vi "Meas Process Config Panel.vi"(8 "error in (no error)":errorcluster, 11 "session in":T4={"adc"={"niScope"={"channel cfg"=[], "sessions"=[], "multi cards"=FALSE, "channels"=0, "type"=enum."n/a", "memory [B/chn]"=0, "ext. clock [Hz]"=0.0, "samples count"=0, "use streaming"=FALSE, "proc setup"={"packet size [smpl]"=0, "current timeout [s]"=0.0, "blk2blk timeout [s]"=0.0, "event time"=timestamp(0 s since 1904-01-01), "temp sampl T [s]"=0.0, "data queue"=refnum, "stop notifier"=refnum, "proc ref"=refnum}, "sample width [B]"=0, "ranges [V]"=[], "trigger setup"={"coupling"=1, "level [V]"=0.0, "slope"=0, "mode"=enum."Immediate", "pre-trigger [%]"=0.0}, "fs [Hz]"=0.0, "bitres [bit]"=0, "clock source"=enum."VAL_NO_SOURCE"}, "3458A"={"channels"=[], "sync unit"={"VISA"="", "type"=enum."Picotest U6200A"}, "awg unit"={"type"=enum."Agilent 331xxA to 332xxA", "VISA"="", "enable 10MHz ref"=FALSE, "cmi ckd2"={"VISA"="", "clock source"=enum."Auto", "manual ref clk"=FALSE, "ref clock [Hz]"=0.0, "div mode"=enum."Set divisor directly"}, "cmi sync v3"={"VISA"="", "baud rate [bd/s]"=115200, "source"=enum."Auto", "hv range"=enum."1kV", "fsrc is fixed"=FALSE, "fsrc [Hz]"=10000000.0, "freq integ [s]"=1.0, "freq filter"=5, "trig level"=enum."TTL 5V", "chn1 mode"=enum."Source divider", "chn1 level"=enum."Positive 5V", "chn2 mode"=enum."Source divider", "chn2 level"=enum."Positive 5V", "chn2 div"=1, "chn3 mode"=enum."Chn 1 Active", "chn3 level"=enum."Positive 5V", "chn1 div entry"=enum."Calculate nearest divisor from measured fx", "chn1 dev limit [%]"=1.0, "chn1 check dev"=FALSE}, "trigger"={"source"=enum."Immediate", "slope"=enum."POS", "coupling"=enum."DC", "level [V]"=0.0, "hysteresis [V]"=0.0, "pre-trigger [%]"=0.0}, "HMF2500 cfg"={"Baud Rate"=9600, "Parity"=0, "Data Bits"=8, "Flow Control"=4}}, "sync mode"=enum."MASTER-SLAVE, MASTER clocked by TIMER", "streaming mode"=FALSE, "idn mode"=enum."Auto", "sampling mode"=enum."DCV", "sample memory [B]"=0, "proc setup"={"channel id"=0, "packet size [smpl]"=0, "current timeout [s]"=0.0, "blk2blk timeout [s]"=0.0, "event time"=timestamp(0 s since 1904-01-01), "stop notifier"=refnum, "data queues"=[], "proc refs"=[], "bus semaphore"=refnum}, "sample size [B]"=0, "sample count"=0, "aux data"={"channel id"=0, "valid?"=[], "gain [V]"=[], "timestamp [s]"=[], "Ts [s]"=0.0, "abs timestamp"=timestamp(0 s since 1904-01-01), "t [deg C]"=[], "multiplex timestamp [s]"=-1.0, "only multiplex?"=FALSE, "multiplex smpl offset"=0, "overflow?"=FALSE}, "ranges [V]"=[], "aperture [s]"=0.0, "LEVEL trigger"={"edge"=enum."POS", "level [V]"=0.0, "coupling"=enum."DC"}, "trigger mode"=enum."AUTO", "measure temp.?"=FALSE, "disp mesages"=[], "shared bus?"=FALSE, "disable display?"=FALSE, "aper mode"=enum."Manual", "aper rules"=[], "multiplex"={"cycles"=0, "delay [s]"=0.0, "enabled"=FALSE, "overhead [s]"=1.0, "tot smpls"=0, "sub-rec"=0, "overhead [%]"=0.0, "emulated"=FALSE}, "F8588 lpf"=enum."Off", "F8588 pll"=enum."Off", "F8588 couple"=enum."DC, auto", "fs"={"freq mode"=enum."fs or Ts", "fs [Hz]"=0.0, "fref [Hz]"=0.0, "mul"=0.0, "div"=0.0}, "fs mode"=enum."fs or Ts", "init timestamp"=timestamp(0 s since 1904-01-01), "last report timestamp"=timestamp(0 s since 1904-01-01)}, "dsdll"={"dsdll"={"dsdll path"=path "", "dsdll handle"=[], "output devices"=[], "capture devices"=[]}, "channels"=0, "device id"=0, "channel idns"=[], "proc setup"={"packet size [smpl]"=0, "current timeout [s]"=0.0, "blk2blk timeout [s]"=0.0, "event time"=timestamp(0 s since 1904-01-01), "data queue"=refnum, "stop notifier"=refnum, "proc ref"=refnum}, "samples count"=0, "fs [Hz]"=0.0}, "type"=enum."niScope", "channel idn str"=[], "aux instr idn str"=[], "modified?"=FALSE, "simadc"={"channels"=[], "range [V]"=0.0, "Ts step [s]"=0.0, "time [s]"=0.0, "fs [Hz]"=0.0, "count"=0, "smpl offset"=0, "set count"=0, "bit res"=0}, "force rst?"=FALSE, "exit mode"=enum."Immediate reset", "exit dly"=0.0, "exit tmr"=timestamp(0 s since 1904-01-01), "busy?"=FALSE, "accessed?"=FALSE, "multiplex"={"Type"=enum."Dummy", "gen com ssn"={"visa"="", "primary"=enum."None", "secondary"=enum."None", "channels"=[]}, "delay before [s]"=0.0, "delay post [s]"=0.0, "sequence"=[], "enabled"=FALSE, "ref timestamp [s]"=0.0, "idn string"="", "dev niScope"="", "niScope idx"=0, "QPMX ssn"={"visa"="", "switch mode"=enum."Switched by TWM", "sequence"=[], "timing delays"=[], "polarity"=enum."Positive", "ss delay (s)"=2.0, "internal timer (s)"=1.0, "Last loaded sequence file"=path "", "startup delay (s)"=2.0}, "VISA mux ssn"={"VISA"="", "paths"=[], "idn command"="", "serial cfg"={"Baud rate"=9600, "Data bits"=8, "Parity"=0, "Stop bits"=10, "Flow control"=0, "End Mode Read"=enum."None", "End Mode Write"=enum."None", "Term character"=0, "Term enable"=FALSE}}}, "keysight dso"={"VISA"="", "channels"=[], "bw limit [Hz]"=0.0, "resolution"=enum."Basic", "trig noise reject"=enum."Normal", "N"=0, "trigger config"={"trigger source"=enum."Immediate", "trigger slope"=enum."Negative", "level [V]"=0.0, "hysteresis [V]"=0.001, "pre-trig [%]"=50}, "fs [Hz]"=0.0, "timeout stop"=timestamp(0 s since 1904-01-01), "waiting for opc"=FALSE, "fetch offset [smpl]"=0, "abs timestamp"=timestamp(0 s since 1904-01-01), "ranges [V]"=[], "decimation"=1.0, "ext ref"=FALSE, "emulate aperture"=FALSE, "model"=enum."DSO91304"}, "cdaq"={"mclk [Hz]"=12800000.0, "ADC task"="", "mclk reference"="", "fs [Hz]"=50000.0, "queue adc cmd"=refnum, "queue adc data"=refnum, "adc proc ref"=refnum, "channels"=[], "last channels"=[], "timeout"=timestamp(0 s since 1904-01-01), "N"=1000, "mclk mode"=enum."Free running", "ext mclk source"=""}, "ignore overload"=FALSE, "ADS127L21"={"VISA"="", "chn list"=[], "record size"=0, "phys. channels"=0, "adc fifo size"=0, "channels"=[], "ext refclk?"=FALSE, "fs [Hz]"=0.0, "ext refclk [Hz]"=0.0, "meas refclk [Hz]"=0.0, "EXTOUT mode"=enum."ADCCLK", "EXTOUT polarity"=enum."NORM", "EXTOUT divisor"=0}}, "sequence"=[], "sequence setup"={"group setups"=[], "rec count"=0, "range mode"=enum."Keep defaults", "fs mode"=enum."Frequency", "rng even"=0.0, "rng odd"=0.0, "folder"=path "", "name base"="", "meas id"=0, "settle [s]"=0.0, "comment"="", "avg count"=0, "fs-abs-fr fr"=0.0, "fs-abs-fr fs"=0.0, "fs-div fr"=0.0, "fs-div div"=0.0, "fs-mn fr"=0.0, "fs-mn mul"=0.0, "fs-mn div"=0.0, "fs-rat fr"=0.0, "fs-rat rat"=0.0}, "golpi"=refnum, "processing setup"={"mode"=enum."Raw", "call after avgs?"=FALSE, "calculate?"=FALSE, "raw mode"={"command"="", "result mode"=enum."Display console output (only Octave)", "res variable"=""}, "QWTB"={"QWTB path"=path "", "alg filter path"="", "alg ids"=[], "alg parameters"=[], "parsed parameters"=[], "selected alg id"="", "selected unc mode"=enum."None", "qwtb mcc"=100, "qwtb timeout"=90, "qwtb covg"=95.0, "qwtb ofs"=0, "qwtb lim data"=0, "multicore"={"jobs folder"=path "", "cores"=0, "max jobs"=0, "mode"=enum."Singlecore"}, "unc once?"=FALSE, "qwtb tstemp"=enum."Enabled (default)", "octave reset"=FALSE, "exec mode"=enum."Single-core"}}, "corrections"={"transducers"={"channels"=[], "last path"=path "", "root path"=path ""}, "digitizer"={"last path"=path "", "channel paths"=[], "channel idns"=[], "correction name"="", "channel names"=[], "folders to copy"=[], "channel valid"=[], "correction path"=path "", "correction rel path"="", "rel folders to copy"=[], "root path"=path ""}}, "assist cfg"={"P"=0, "Q"=0, "rel shift"=0.0, "ref freq"=0.0, "min fs"=0.0, "max fs tol"=0.0, "min int"=0.0, "max int"=0.0, "max err"=0.0, "max timeout"=0.0}} {"corrections"."transducers"."channels"."Phase index" min=1 step=1; "adc"."ADS127L21"."channels"."Channel" min=1 max=8 step=1; "adc"."ADS127L21"."channels"."Range [Vpk]" items=["±1.65V", "±2V"]; "adc"."cdaq"."last channels"."Channel id" min=0 step=1; "adc"."cdaq"."channels"."Channel id" min=0 step=1; "adc"."keysight dso"."decimation" min=1.0; "adc"."keysight dso"."bw limit [Hz]" format="%#_6p"; "adc"."keysight dso"."channels"."Offset [V]" format="%#_6p"; "adc"."keysight dso"."channels"."Range [Vpk]" min=0.0 format="%#_6p"; "adc"."keysight dso"."channels"."Channel" min=1; "adc"."multiplex"."VISA mux ssn"."serial cfg"."Flow control" items=["None", "XON/XOFF", "CTS/RTS", "XON/XOFF + CTS/RTS", "DTR/DSR", "XON/XOFF + DTR/DSR"]; "adc"."multiplex"."VISA mux ssn"."serial cfg"."Stop bits" items=["1 bit"=10, "1.5 bits"=15, "2 bits"=20]; "adc"."multiplex"."VISA mux ssn"."serial cfg"."Parity" items=["None", "Odd", "Even", "Mark", "Space"]; "adc"."multiplex"."VISA mux ssn"."serial cfg"."Data bits" items=["5 bits"=5, "6 bits"=6, "7 bits"=7, "8 bits"=8]; "adc"."multiplex"."VISA mux ssn"."serial cfg"."Baud rate" items=["150 Bd"=150, "300 Bd"=300, "600 Bd"=600, "1200 Bd"=1200, "2400 Bd"=2400, "4800 Bd"=4800, "9600 Bd"=9600, "19.2 kBd"=19200, "38.4 kBd"=38400, "57.6 kBd"=57600, "115.2 kBd"=115200]; "adc"."multiplex"."QPMX ssn"."startup delay (s)" min=0.0 step=1.0; "adc"."multiplex"."QPMX ssn"."internal timer (s)" min=0.0 step=1.0; "adc"."multiplex"."QPMX ssn"."ss delay (s)" min=0.0 step=1.0; "adc"."multiplex"."QPMX ssn"."timing delays" min=1 max=255 step=1; "adc"."3458A"."awg unit"."HMF2500 cfg"."Flow Control" items=["None", "XON/XOFF", "RTS/CTS", "XON/XOFF & RTS/CTS", "DTR/DSR", "XON/XOFF & DTR/DSR"]; "adc"."3458A"."awg unit"."HMF2500 cfg"."Data Bits" items=["7"=7, "8"=8]; "adc"."3458A"."awg unit"."HMF2500 cfg"."Parity" items=["None", "Odd", "Even", "Mark", "Space"]; "adc"."3458A"."awg unit"."HMF2500 cfg"."Baud Rate" items=["300"=300, "600"=600, "1200"=1200, "2400"=2400, "4800"=4800, "9600"=9600, "19200"=19200]; "adc"."3458A"."awg unit"."cmi sync v3"."chn2 div" min=1 max=100000000 step=1; "adc"."3458A"."awg unit"."cmi sync v3"."fsrc [Hz]" format="%_8p"; "adc"."3458A"."channels"."Range [Vpk]" min=0.0; "adc"."niScope"."trigger setup"."pre-trigger [%]" format="%.2f"; "adc"."niScope"."trigger setup"."level [V]" format="%.2f"; "adc"."niScope"."trigger setup"."coupling" items=["AC"=0, "DC"=1, "HF Reject"=3, "LF Reject"=4, "AC Plus HF Reject"=1001]; "adc"."niScope"."channel cfg"."Range [Vpk]" min=0.0; "adc"."niScope"."channel cfg"."Channel" min=0}) -> (0 "error out":errorcluster, 3 "session out":T4={"adc"={"niScope"={"channel cfg"=[], "sessions"=[], "multi cards"=FALSE, "channels"=0, "type"=enum."n/a", "memory [B/chn]"=0, "ext. clock [Hz]"=0.0, "samples count"=0, "use streaming"=FALSE, "proc setup"={"packet size [smpl]"=0, "current timeout [s]"=0.0, "blk2blk timeout [s]"=0.0, "event time"=timestamp(0 s since 1904-01-01), "temp sampl T [s]"=0.0, "data queue"=refnum, "stop notifier"=refnum, "proc ref"=refnum}, "sample width [B]"=0, "ranges [V]"=[], "trigger setup"={"coupling"=1, "level [V]"=0.0, "slope"=0, "mode"=enum."Immediate", "pre-trigger [%]"=0.0}, "fs [Hz]"=0.0, "bitres [bit]"=0, "clock source"=enum."VAL_NO_SOURCE"}, "3458A"={"channels"=[], "sync unit"={"VISA"="", "type"=enum."Picotest U6200A"}, "awg unit"={"type"=enum."Agilent 331xxA to 332xxA", "VISA"="", "enable 10MHz ref"=FALSE, "cmi ckd2"={"VISA"="", "clock source"=enum."Auto", "manual ref clk"=FALSE, "ref clock [Hz]"=0.0, "div mode"=enum."Set divisor directly"}, "cmi sync v3"={"VISA"="", "baud rate [bd/s]"=115200, "source"=enum."Auto", "hv range"=enum."1kV", "fsrc is fixed"=FALSE, "fsrc [Hz]"=10000000.0, "freq integ [s]"=1.0, "freq filter"=5, "trig level"=enum."TTL 5V", "chn1 mode"=enum."Source divider", "chn1 level"=enum."Positive 5V", "chn2 mode"=enum."Source divider", "chn2 level"=enum."Positive 5V", "chn2 div"=1, "chn3 mode"=enum."Chn 1 Active", "chn3 level"=enum."Positive 5V", "chn1 div entry"=enum."Calculate nearest divisor from measured fx", "chn1 dev limit [%]"=1.0, "chn1 check dev"=FALSE}, "trigger"={"source"=enum."Immediate", "slope"=enum."POS", "coupling"=enum."DC", "level [V]"=0.0, "hysteresis [V]"=0.0, "pre-trigger [%]"=0.0}, "HMF2500 cfg"={"Baud Rate"=9600, "Parity"=0, "Data Bits"=8, "Flow Control"=4}}, "sync mode"=enum."MASTER-SLAVE, MASTER clocked by TIMER", "streaming mode"=FALSE, "idn mode"=enum."Auto", "sampling mode"=enum."DCV", "sample memory [B]"=0, "proc setup"={"channel id"=0, "packet size [smpl]"=0, "current timeout [s]"=0.0, "blk2blk timeout [s]"=0.0, "event time"=timestamp(0 s since 1904-01-01), "stop notifier"=refnum, "data queues"=[], "proc refs"=[], "bus semaphore"=refnum}, "sample size [B]"=0, "sample count"=0, "aux data"={"channel id"=0, "valid?"=[], "gain [V]"=[], "timestamp [s]"=[], "Ts [s]"=0.0, "abs timestamp"=timestamp(0 s since 1904-01-01), "t [deg C]"=[], "multiplex timestamp [s]"=-1.0, "only multiplex?"=FALSE, "multiplex smpl offset"=0, "overflow?"=FALSE}, "ranges [V]"=[], "aperture [s]"=0.0, "LEVEL trigger"={"edge"=enum."POS", "level [V]"=0.0, "coupling"=enum."DC"}, "trigger mode"=enum."AUTO", "measure temp.?"=FALSE, "disp mesages"=[], "shared bus?"=FALSE, "disable display?"=FALSE, "aper mode"=enum."Manual", "aper rules"=[], "multiplex"={"cycles"=0, "delay [s]"=0.0, "enabled"=FALSE, "overhead [s]"=1.0, "tot smpls"=0, "sub-rec"=0, "overhead [%]"=0.0, "emulated"=FALSE}, "F8588 lpf"=enum."Off", "F8588 pll"=enum."Off", "F8588 couple"=enum."DC, auto", "fs"={"freq mode"=enum."fs or Ts", "fs [Hz]"=0.0, "fref [Hz]"=0.0, "mul"=0.0, "div"=0.0}, "fs mode"=enum."fs or Ts", "init timestamp"=timestamp(0 s since 1904-01-01), "last report timestamp"=timestamp(0 s since 1904-01-01)}, "dsdll"={"dsdll"={"dsdll path"=path "", "dsdll handle"=[], "output devices"=[], "capture devices"=[]}, "channels"=0, "device id"=0, "channel idns"=[], "proc setup"={"packet size [smpl]"=0, "current timeout [s]"=0.0, "blk2blk timeout [s]"=0.0, "event time"=timestamp(0 s since 1904-01-01), "data queue"=refnum, "stop notifier"=refnum, "proc ref"=refnum}, "samples count"=0, "fs [Hz]"=0.0}, "type"=enum."niScope", "channel idn str"=[], "aux instr idn str"=[], "modified?"=FALSE, "simadc"={"channels"=[], "range [V]"=0.0, "Ts step [s]"=0.0, "time [s]"=0.0, "fs [Hz]"=0.0, "count"=0, "smpl offset"=0, "set count"=0, "bit res"=0}, "force rst?"=FALSE, "exit mode"=enum."Immediate reset", "exit dly"=0.0, "exit tmr"=timestamp(0 s since 1904-01-01), "busy?"=FALSE, "accessed?"=FALSE, "multiplex"={"Type"=enum."Dummy", "gen com ssn"={"visa"="", "primary"=enum."None", "secondary"=enum."None", "channels"=[]}, "delay before [s]"=0.0, "delay post [s]"=0.0, "sequence"=[], "enabled"=FALSE, "ref timestamp [s]"=0.0, "idn string"="", "dev niScope"="", "niScope idx"=0, "QPMX ssn"={"visa"="", "switch mode"=enum."Switched by TWM", "sequence"=[], "timing delays"=[], "polarity"=enum."Positive", "ss delay (s)"=2.0, "internal timer (s)"=1.0, "Last loaded sequence file"=path "", "startup delay (s)"=2.0}, "VISA mux ssn"={"VISA"="", "paths"=[], "idn command"="", "serial cfg"={"Baud rate"=9600, "Data bits"=8, "Parity"=0, "Stop bits"=10, "Flow control"=0, "End Mode Read"=enum."None", "End Mode Write"=enum."None", "Term character"=0, "Term enable"=FALSE}}}, "keysight dso"={"VISA"="", "channels"=[], "bw limit [Hz]"=0.0, "resolution"=enum."Basic", "trig noise reject"=enum."Normal", "N"=0, "trigger config"={"trigger source"=enum."Immediate", "trigger slope"=enum."Negative", "level [V]"=0.0, "hysteresis [V]"=0.001, "pre-trig [%]"=50}, "fs [Hz]"=0.0, "timeout stop"=timestamp(0 s since 1904-01-01), "waiting for opc"=FALSE, "fetch offset [smpl]"=0, "abs timestamp"=timestamp(0 s since 1904-01-01), "ranges [V]"=[], "decimation"=1.0, "ext ref"=FALSE, "emulate aperture"=FALSE, "model"=enum."DSO91304"}, "cdaq"={"mclk [Hz]"=12800000.0, "ADC task"="", "mclk reference"="", "fs [Hz]"=50000.0, "queue adc cmd"=refnum, "queue adc data"=refnum, "adc proc ref"=refnum, "channels"=[], "last channels"=[], "timeout"=timestamp(0 s since 1904-01-01), "N"=1000, "mclk mode"=enum."Free running", "ext mclk source"=""}, "ignore overload"=FALSE, "ADS127L21"={"VISA"="", "chn list"=[], "record size"=0, "phys. channels"=0, "adc fifo size"=0, "channels"=[], "ext refclk?"=FALSE, "fs [Hz]"=0.0, "ext refclk [Hz]"=0.0, "meas refclk [Hz]"=0.0, "EXTOUT mode"=enum."ADCCLK", "EXTOUT polarity"=enum."NORM", "EXTOUT divisor"=0}}, "sequence"=[], "sequence setup"={"group setups"=[], "rec count"=0, "range mode"=enum."Keep defaults", "fs mode"=enum."Frequency", "rng even"=0.0, "rng odd"=0.0, "folder"=path "", "name base"="", "meas id"=0, "settle [s]"=0.0, "comment"="", "avg count"=0, "fs-abs-fr fr"=0.0, "fs-abs-fr fs"=0.0, "fs-div fr"=0.0, "fs-div div"=0.0, "fs-mn fr"=0.0, "fs-mn mul"=0.0, "fs-mn div"=0.0, "fs-rat fr"=0.0, "fs-rat rat"=0.0}, "golpi"=refnum, "processing setup"={"mode"=enum."Raw", "call after avgs?"=FALSE, "calculate?"=FALSE, "raw mode"={"command"="", "result mode"=enum."Display console output (only Octave)", "res variable"=""}, "QWTB"={"QWTB path"=path "", "alg filter path"="", "alg ids"=[], "alg parameters"=[], "parsed parameters"=[], "selected alg id"="", "selected unc mode"=enum."None", "qwtb mcc"=100, "qwtb timeout"=90, "qwtb covg"=95.0, "qwtb ofs"=0, "qwtb lim data"=0, "multicore"={"jobs folder"=path "", "cores"=0, "max jobs"=0, "mode"=enum."Singlecore"}, "unc once?"=FALSE, "qwtb tstemp"=enum."Enabled (default)", "octave reset"=FALSE, "exec mode"=enum."Single-core"}}, "corrections"={"transducers"={"channels"=[], "last path"=path "", "root path"=path ""}, "digitizer"={"last path"=path "", "channel paths"=[], "channel idns"=[], "correction name"="", "channel names"=[], "folders to copy"=[], "channel valid"=[], "correction path"=path "", "correction rel path"="", "rel folders to copy"=[], "root path"=path ""}}, "assist cfg"={"P"=0, "Q"=0, "rel shift"=0.0, "ref freq"=0.0, "min fs"=0.0, "max fs tol"=0.0, "min int"=0.0, "max int"=0.0, "max err"=0.0, "max timeout"=0.0}} {"corrections"."transducers"."channels"."Phase index" min=1 step=1; "adc"."ADS127L21"."channels"."Channel" min=1 max=8 step=1; "adc"."ADS127L21"."channels"."Range [Vpk]" items=["±1.65V", "±2V"]; "adc"."cdaq"."last channels"."Channel id" min=0 step=1; "adc"."cdaq"."channels"."Channel id" min=0 step=1; "adc"."keysight dso"."decimation" min=1.0; "adc"."keysight dso"."bw limit [Hz]" format="%#_6p"; "adc"."keysight dso"."channels"."Offset [V]" format="%#_6p"; "adc"."keysight dso"."channels"."Range [Vpk]" min=0.0 format="%#_6p"; "adc"."keysight dso"."channels"."Channel" min=1; "adc"."multiplex"."VISA mux ssn"."serial cfg"."Flow control" items=["None", "XON/XOFF", "CTS/RTS", "XON/XOFF + CTS/RTS", "DTR/DSR", "XON/XOFF + DTR/DSR"]; "adc"."multiplex"."VISA mux ssn"."serial cfg"."Stop bits" items=["1 bit"=10, "1.5 bits"=15, "2 bits"=20]; "adc"."multiplex"."VISA mux ssn"."serial cfg"."Parity" items=["None", "Odd", "Even", "Mark", "Space"]; "adc"."multiplex"."VISA mux ssn"."serial cfg"."Data bits" items=["5 bits"=5, "6 bits"=6, "7 bits"=7, "8 bits"=8]; "adc"."multiplex"."VISA mux ssn"."serial cfg"."Baud rate" items=["150 Bd"=150, "300 Bd"=300, "600 Bd"=600, "1200 Bd"=1200, "2400 Bd"=2400, "4800 Bd"=4800, "9600 Bd"=9600, "19.2 kBd"=19200, "38.4 kBd"=38400, "57.6 kBd"=57600, "115.2 kBd"=115200]; "adc"."multiplex"."QPMX ssn"."startup delay (s)" min=0.0 step=1.0; "adc"."multiplex"."QPMX ssn"."internal timer (s)" min=0.0 step=1.0; "adc"."multiplex"."QPMX ssn"."ss delay (s)" min=0.0 step=1.0; "adc"."multiplex"."QPMX ssn"."timing delays" min=1 max=255 step=1; "adc"."3458A"."awg unit"."HMF2500 cfg"."Flow Control" items=["None", "XON/XOFF", "RTS/CTS", "XON/XOFF & RTS/CTS", "DTR/DSR", "XON/XOFF & DTR/DSR"]; "adc"."3458A"."awg unit"."HMF2500 cfg"."Data Bits" items=["7"=7, "8"=8]; "adc"."3458A"."awg unit"."HMF2500 cfg"."Parity" items=["None", "Odd", "Even", "Mark", "Space"]; "adc"."3458A"."awg unit"."HMF2500 cfg"."Baud Rate" items=["300"=300, "600"=600, "1200"=1200, "2400"=2400, "4800"=4800, "9600"=9600, "19200"=19200]; "adc"."3458A"."awg unit"."cmi sync v3"."chn2 div" min=1 max=100000000 step=1; "adc"."3458A"."awg unit"."cmi sync v3"."fsrc [Hz]" format="%_8p"; "adc"."3458A"."channels"."Range [Vpk]" min=0.0; "adc"."niScope"."trigger setup"."pre-trigger [%]" format="%.2f"; "adc"."niScope"."trigger setup"."level [V]" format="%.2f"; "adc"."niScope"."trigger setup"."coupling" items=["AC"=0, "DC"=1, "HF Reject"=3, "LF Reject"=4, "AC Plus HF Reject"=1001]; "adc"."niScope"."channel cfg"."Range [Vpk]" min=0.0; "adc"."niScope"."channel cfg"."Channel" min=0})   [LabVIEW 2020]
doc: "Configuration panel for result calculator. Select tab to select method of calculation."
uses:
  Meas Session.ctl
  adc/ADC Session.ctl
  drivers/niScope/niScope Session.ctl
  drivers/niScope/niScope Virtual Channel Config.ctl
  drivers/niScope/niScope Virtual Channel Mode.ctl
  drivers/niScope/niScope Virtual Channel Input Z.ctl
  drivers/niScope/niScope Virtual Channel Coupling.ctl
  drivers/niScope/niScope Type.ctl
  drivers/niScope/niScope Digitizing Process Options.ctl
  drivers/niScope/niScope Data Packet.ctl
  drivers/niScope/niScope Trigger Setup.ctl
  <instrlib>/niScope/Controls/niScope trigger coupling.ctl
  <instrlib>/niScope/Controls/niScope trigger slope.ctl
  drivers/niScope/niScope Reference Clock.ctl
  drivers/DMM/3458A Digitizer Session.ctl
  drivers/DMM/3458A Virtual Channel Config.ctl
  drivers/Counter/Counter Session.ctl
  drivers/Counter/Counter Type.ctl
  drivers/AWG/AWG Session.ctl
  drivers/AWG/AWG Type.ctl
  drivers/AWG/CMI Clock Divider v2/CMI ckd2 Session.ctl
  drivers/AWG/CMI Clock Divider v2/CMI ckd2 Source Mode.ctl
  drivers/AWG/CMI Clock Divider v2/CMI ckd2 Divisor Mode.ctl
  drivers/AWG/CMI Sync V3/CMI Sync V3 session.ctl
  drivers/AWG/CMI Sync V3/Configure/CMI Sync V3 Reference Clock Source.ctl
  drivers/AWG/CMI Sync V3/Configure/CMI Sync V3 HV input Range.ctl
  drivers/AWG/CMI Sync V3/Configure/CMI Sync V3 Trigger Input Level.ctl
  drivers/AWG/CMI Sync V3/Configure/CMI Sync V3 Channel 1 Mode.ctl
  drivers/AWG/CMI Sync V3/Configure/CMI Sync V3 Channel Output Levels.ctl
  drivers/AWG/CMI Sync V3/Configure/CMI Sync V3 Channel 2 Mode.ctl
  drivers/AWG/CMI Sync V3/Configure/CMI Sync V3 Channel 3 Mode.ctl
  drivers/AWG/CMI Sync V3/Configure/CMI Sync V3 Channel 1 Divisor Entry Mode.ctl
  adc/ADC Trig Config.ctl
  adc/ADC Trig Mode Source.ctl
  adc/ADC Trig Slope.ctl
  adc/ADC Trig Coupling.ctl
  drivers/AWG/RaS HMF2500/HMF2500 Config.ctl
  drivers/DMM/3458A Sync Mode.ctl
  drivers/DMM/3458A Idn Mode.ctl
  drivers/DMM/3458A Digitizing Low Levels/Configure/Sampling Mode.ctl
  drivers/DMM/3458A Digitizing Process Options.ctl
  drivers/DMM/3458A Data Packet.ctl
  drivers/DMM/3458A Aux Record Data.ctl
  drivers/DMM/3458A Digitizing Low Levels/Configure/Level Setup.ctl
  drivers/DMM/3458A Digitizing Low Levels/Configure/First Sample Trigger.ctl
  drivers/DMM/3458A Aperture Selection Mode.ctl
  drivers/DMM/3458A Multiplexing Config.ctl
  drivers/Fluke 8588A/F8588A Low Pass Filter.ctl
  drivers/Fluke 8588A/F8588A Phase Lock.ctl
  drivers/Fluke 8588A/F8588A Coupling.ctl
  drivers/DMM/3458A Sampling Rate.ctl
  drivers/AWG/AWG Clock Setup Mode.ctl
  drivers/DMM/3458A Sample Rate Mode.ctl
  drivers/dsdll/DSDLL Session.ctl
  drivers/dsdll/dsdll/dsdll_instance.ctl
  drivers/dsdll/dsdll/dsdll_device_record.ctl
  drivers/dsdll/DSDLL Process Config.ctl
  drivers/dsdll/DSDLL Data Packet.ctl
  adc/ADC Type.ctl
  drivers/simulated_adc/SimAdc Config.ctl
  drivers/simulated_adc/SimAdc Channel Cfg.ctl
  adc/ADC On Close Action.ctl
  adc/Multiplexer/MPX Session.ctl
  adc/Multiplexer/MPX Type.ctl
  drivers/Multiplexers/Generic COM/GCOMM Session.ctl
  drivers/Multiplexers/Generic COM/GCOMM Signal.ctl
  drivers/Multiplexers/Generic COM/GCOMM Virtual Channel.ctl
  drivers/Multiplexers/Generic COM/GCOMM Logic State.ctl
  drivers/Multiplexers/Generic COM/QPMX Session.ctl
  drivers/Multiplexers/QPMX/QPMX switch mode.ctl
  drivers/Multiplexers/QPMX/QPMX polarity.ctl
  drivers/Multiplexers/Generic VISA commands/GVISA Mux Session.ctl
  drivers/Multiplexers/Generic VISA commands/GVISA Mux Path Entry.ctl
  drivers/Multiplexers/Generic VISA commands/met_serial_setup.ctl
  drivers/Agilent DSO 90000/Virtual Digitizer/KeDSO session.ctl
  drivers/Agilent DSO 90000/Virtual Digitizer/KeDSO Virtual Channel.ctl
  drivers/Agilent DSO 90000/Virtual Digitizer/KeDSO High Resolution Mode.ctl
  drivers/Agilent DSO 90000/Virtual Digitizer/KeDSO Trigger Setup.ctl
  drivers/Agilent DSO 90000/Virtual Digitizer/KeDSO Trigger Source.ctl
  drivers/Agilent DSO 90000/Public/Utility/DSO type.ctl
  drivers/cdaq/cDAQ Session.ctl
  drivers/cdaq/low_level_old/cdaq_anal_adc_command.ctl
  drivers/cdaq/low_level_old/cdaq_anal_adc_data.ctl
  drivers/cdaq/cDAQ Virtual Channel.ctl
  drivers/cdaq/cDAQ Master Clock Mode.ctl
  drivers/CMI_ADS127L21/CMI ADS127L21 - Session.ctl
  drivers/CMI_ADS127L21/CMI ADS127L21 - Record Channel.ctl
  drivers/CMI_ADS127L21/CMI ADS127L21 - Input Range.ctl
  drivers/CMI_ADS127L21/CMI ADS127L21 - Input Mode.ctl
  drivers/CMI_ADS127L21/CMI ADS127L21 - Input Impedance.ctl
  drivers/CMI_ADS127L21/CMI ADS127L21 - EXTOUT Mode.ctl
  drivers/CMI_ADS127L21/CMI ADS127L21 - EXTOUT Polarity.ctl
  Meas Sequence Item.ctl
  Meas Sampling Configuration.ctl
  QWTB/Meas Proc QWTB Algorithm Parameter Data.ctl
  Meas Sequence Configuration.ctl
  Meas Range Mode.ctl
  Meas Sampling Rate Mode.ctl
  octave/golpi/mpc/golpi_session_ref.ctl
  octave/golpi/mpc/golpi_session.ctl
  octave/golpi/GOLPI reference Type Def.ctl
  octave/golpi/Pipe Handle.ctl
  Meas Process Config.ctl
  Meas Process Mode.ctl
  Meas Process Raw Config.ctl
  Meas Process Raw Result Mode.ctl
  QWTB/Meas Proc QWTB Setup.ctl
  QWTB/Meas Proc QWTB Uncertainty Mode.ctl
  QWTB/Meas Proc QWTB Multicore Setup.ctl
  QWTB/Meas Proc QWTB Multicore Type.ctl
  Meas Process Time Stamp Mode.ctl
  QWTB/Meas Proc QWTB Exec Mode.ctl
  Corrections/Corr Setup.ctl
  Corrections/Corr Tranducer Item.ctl
  Corrections/Corr Digitizers.ctl
  Assist/Assist Panel Setup.ctl
  varilib/SGUI Assign References Mode.ctl
  varilib/varilib.lvlib
  other/Parameter Matrix/Parameter Matrix Operation.vi
  QWTB/Meas Proc QWTB Quantity Record.ctl
  other/Parameter Matrix/Corr Parameter Item.ctl
  QWTB/Meas Proc QWTB Algorithm Info.ctl
  drivers/niScope/niScope Virtual Digitizer.lvlib
  drivers/DMM/3458A Virtual Digitizer.lvlib
  drivers/Counter/Counter.lvlib
  drivers/AWG/AWG.lvlib
  drivers/DMM/3458A Digitizing Low Levels/3458A Digitizing Low Levels.lvlib
  drivers/dsdll/DSDLL Virtual Digitizer.lvlib
  octave/golpi/mpc/GOLPI Multi Process.lvlib
  drivers/dsdll/dsdll/dsdll.lvlib
  octave/golpi/LV Process library.lvlib
  octave/golpi/GOLPI library.lvlib
  drivers/AWG/CMI Sync V3/CMI Sync Unit V3.lvlib
  drivers/Agilent DSO 90000/Agilent 90000 Series.lvlib
panel:
  out "algorithm info":T1
  in  "btn default":bool
  out "init parameters":bool=TRUE
  in  "btn fake":bool
  in  "btn ok":bool
  in  "tc mode":enum32{"RAW command", "QWTB"}(tab)
  in  "btn raw load m":bool
  in  "raw res var":string caption="Result string variable name"
  in  "raw res mode":T102 caption="Result display mode"
  in  "btn raw example":bool
  in  "raw calc once?":bool caption="Call just once when all averages are done?"
  in  "raw command":string="% load record sample data (path, group id, average id)\ndata = tpq_load_record(%header%, 0, %repid%);\n\n% calculate RMS (for coherent setup)\nrms = sum(data.y.^2,1).^0.5/data.sample_count^0.5\n\n% calculate DC offset (for coherent setup)\ndc = mean(data.y,1)\n\n% calculate spectrum\nN = size(data.y,1);\nU = fft(data.y)*2/N;\nU = U(1:floor(N/2),:)\nfs = [0:floor(N/2)-1]'/data.Ts/N;\n\n% plot it\nloglog(fs,abs(U));" caption="Octave/Matlab command string"
  in  "btn edit qwtb list":bool
  out "qwtb alg can multi":bool caption="Support for multiple records processing"
  in  "qwtb unc once":bool caption="Calculate uncertainty just once?"
  in  "qwtb lim data":bool caption="Limit input data:"
  in  "qwtb lim data size":i64 caption="Input data length [samples]"
  in  "qwtb data ofs":i64 caption="Start offset [sample]"
  in  "qwtb covg":dbl=95.0 caption="Level of Confidence [%]" min=50.0 max=99.99999
  in  "qwtb timeout":i32=90 caption="Processing timeout [s]"
  in  "qwtb mcc":i32=100 caption="Monte-Carlo cycles"
  out "qwtb alg has ui":bool caption="Two inputs algorithm (U and I)"
  out "qwtb alg is diff":bool caption="Supports differential transducer connection"
  in  "qwtb calc once":bool caption="Calculate result just once when all records are measured? (obsolete: use sub-records)"
  in  "qwtb unc mode":T104 caption="Uncertainty calculation mode"
  in  "btn qwtb clr params":bool
  out "qwtb var desc":string caption="Variable description"
  in  "qwtb alg params":string[][](table) caption="Parameters of the algorithm"
  out "qwtb alg cite":string caption="Citation"
  out "qwtb alg note":string caption="Note"
  out "qwtb alg desc":string caption="Description"
  in  "qwtb alg list":u16(ring) caption="List of algorithms" items=["TWM-CLKSKIP: TWM tool wrapper: HP3458A clock skip detector", "TWM-FPNLSF: TWM tool wrapper: Four Parameter Non-Linear Sine Fit", "TWM-Flicker: TWM tool wrapper: Flicker algorithm", "TWM-HCRMS: Half Cycle RMS algorithm", "TWM-InDiSwell: Interruption Dip Swell", "TWM-InpZ: TWM tool wrapper: Input impedance estimator", "TWM-LowZ: TWM tool wrapper: Low impedance measurement algorithm", "TWM-MFSF: Multi Harmonic Frequency Estimator", "TWM-MODTDPS: TWM tool wrapper: Modulation estimator", "TWM-PSFE: TWM tool wrapper: Phase Sensitive Frequency Estimator", "TWM-PWRFFT: Power calculation algorithm using FFT.", "TWM-PWRTDI: Power calculation algorithm using Time-Domain-Integration.", "TWM-PWRTEST: Test/demonstration algorithm for the TWM tool with two inputs", "TWM-RATWFFT: Vector ratio by windowed FFT.", "TWM-TEST: Test/demonstration algorithm for the TWM tool", "TWM-THDWFFT: Harmonic distortion by windowed FFT", "TWM-TIAZ: Impedance measurement using transimpedance amplifier", "TWM-WFFT: Windowed FFT for harmonic analysis.", "TWM-WRMS: RMS level calculation using windowed Time-Domain-Integration."]
  in  "btn load algs":bool
  in  "btn mc cfg":bool
  in  "qwtb tstemp":T107 caption="Time-stamps handling"
  # "ADC:"
  # "ADC:"
  # "Enter Octave command sequence to execute. You can use following variables anywhere in the command sequence:\n\n%header% - full file path of the header file of the current measurement with no extension\n%repid% - id of the current repetition cycle (0 when calculating once after all repetitions are done)\n%respath% - result file path: '%header%-res.info' in the measurement folder"
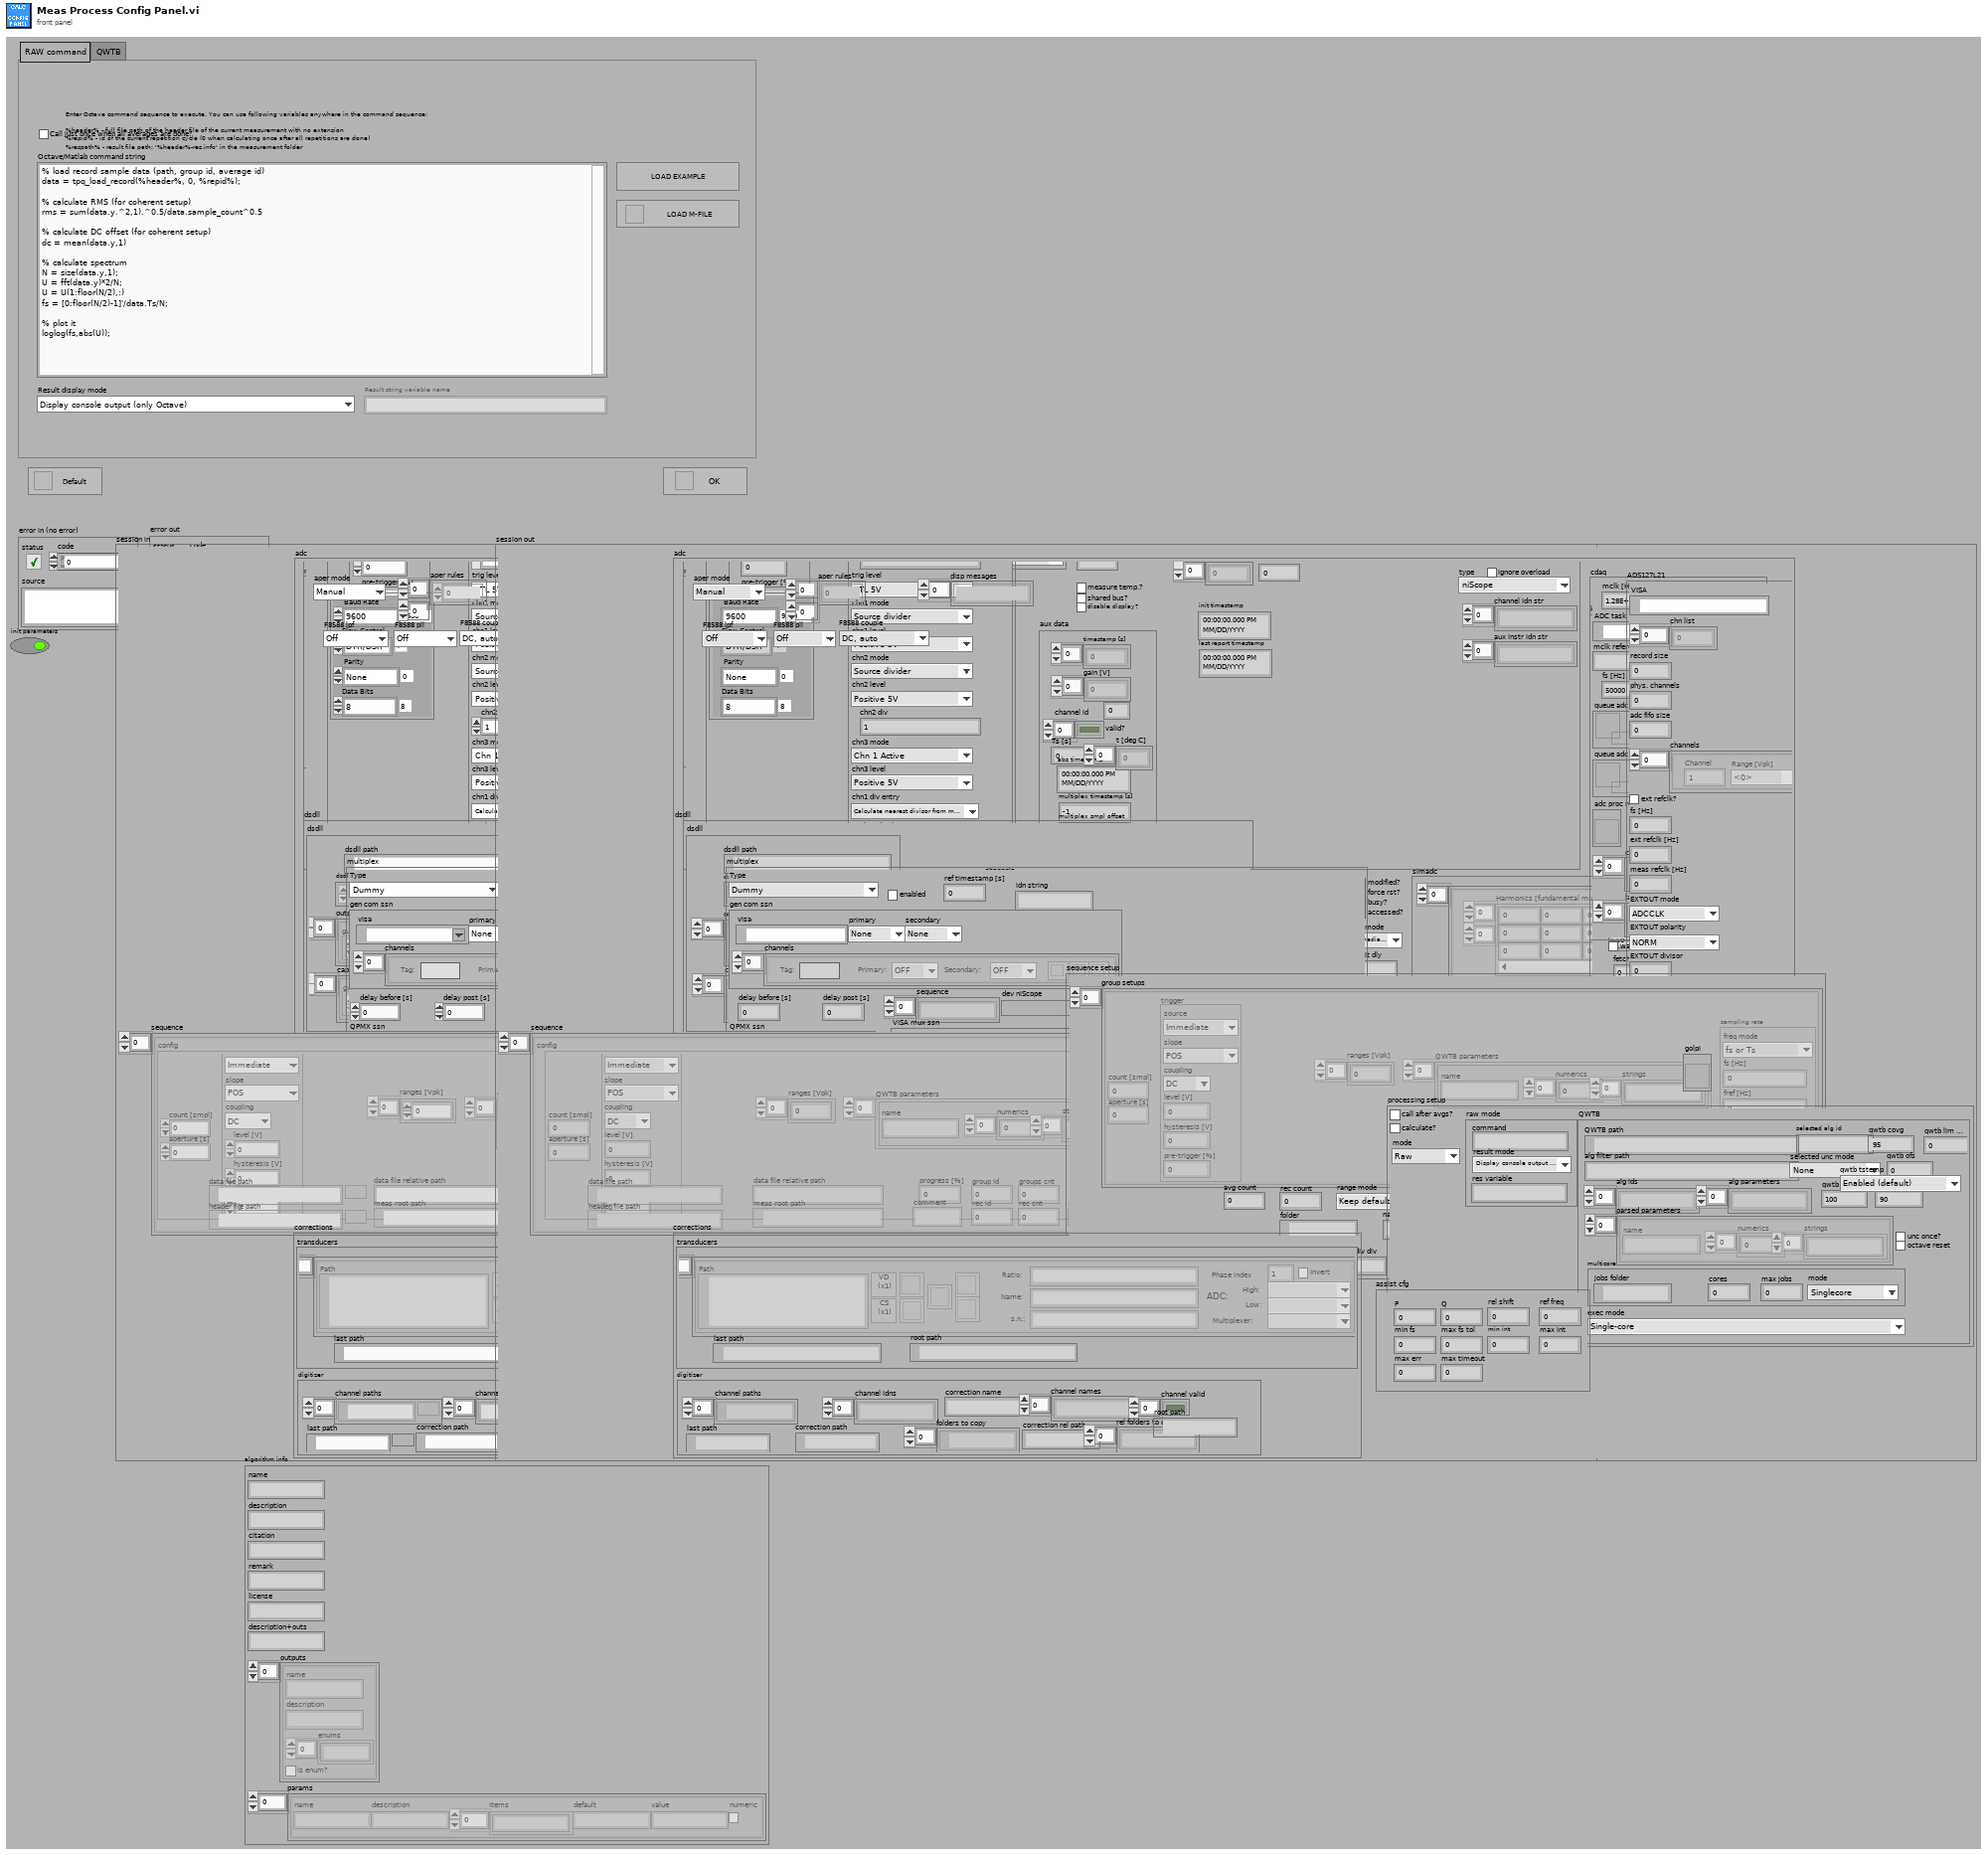
[diagram p1: front panel]
types:
  T1 = typedef "Meas Proc QWTB Algorithm Info.ctl" = cluster{"name":string, "description":string, "citation":string, "remark":string, "license":string, "description+outs":string, "outputs":T2[], "params":T3[]}
  T2 = typedef "Meas Proc QWTB Quantity Record.ctl" = cluster{"name":string, "description":string, "enums":string[], "is enum?":bool}
  T3 = typedef "Corr Parameter Item.ctl" = cluster{"name":string, "description":string, "items":string[], "default":string, "value":string, "numeric":bool}
  T4 = typedef "Meas Session.ctl" = cluster{"adc":T5, "sequence":T92[], "sequence setup":T95, "golpi":T98, "processing setup":T99, "corrections":T109, "assist cfg":T112}
  T5 = typedef "ADC Session.ctl" = cluster{"niScope":T6, "3458A":T17, "dsdll":T56, "type":T60, "channel idn str":string[], "aux instr idn str":string[], "modified?":bool, "simadc":T61, "force rst?":bool, "exit mode":T63, "exit dly":dbl, "exit tmr":timestamp, "busy?":bool, "accessed?":bool, "multiplex":T64, "keysight dso":T76, "cdaq":T82, "ignore overload":bool, "ADS127L21":T85}
  T6 = typedef "niScope Virtual Digitizer.lvlib/niScope Session.ctl" = cluster{"channel cfg":T7[], "sessions":refnum<k20>[], "multi cards":bool, "channels":i32, "type":T11, "memory [B/chn]":i32, "ext. clock [Hz]":dbl, "samples count":i64, "use streaming":bool, "proc setup":T12, "sample width [B]":i32, "ranges [V]":dbl[], "trigger setup":T13, "fs [Hz]":dbl, "bitres [bit]":i32, "clock source":T16}
  T7 = typedef "niScope Virtual Digitizer.lvlib/niScope Virtual Channel Config.ctl" = cluster{"Address":refnum<k15>, "Channel":i32, "Mode":T8, "Input Z":T9, "Coupling":T10, "Range [Vpk]":dbl, "btn clr":bool, "btn up":bool, "btn down":bool}
  T8 = typedef "niScope Virtual Digitizer.lvlib/niScope Virtual Channel Mode.ctl" = enum16{"Single ended", "Unbal. differential", "Differential"}
  T9 = typedef "niScope Virtual Digitizer.lvlib/niScope Virtual Channel Input Z.ctl" = enum16{"1 MOhm", "50 Ohm"}
  T10 = typedef "niScope Virtual Digitizer.lvlib/niScope Virtual Channel Coupling.ctl" = enum16{"AC", "DC", "GND"}
  T11 = typedef "niScope Virtual Digitizer.lvlib/niScope Type.ctl" = enum16{"n/a", "5922"}
  T12 = typedef "niScope Virtual Digitizer.lvlib/niScope Digitizing Process Options.ctl" = cluster{"packet size [smpl]":i64, "current timeout [s]":dbl, "blk2blk timeout [s]":dbl, "event time":timestamp, "temp sampl T [s]":dbl, "data queue":refnum<queue>, "stop notifier":refnum<notifier>, "proc ref":refnum<vi>}
  T13 = typedef "niScope Virtual Digitizer.lvlib/niScope Trigger Setup.ctl" = cluster{"coupling":T14, "level [V]":dbl, "slope":T15, "mode":enum16{"Immediate", "External", "Level"}, "pre-trigger [%]":dbl}
  T14 = typedef "niScope trigger coupling.ctl" = u16
  T15 = typedef "niScope trigger slope.ctl" = i32
  T16 = typedef "niScope Virtual Digitizer.lvlib/niScope Reference Clock.ctl" = enum16{"VAL_NO_SOURCE", "VAL_CLK_IN", "VAL_PXI_CLOCK", "VAL_EXTERNAL"}
  T17 = typedef "3458A Virtual Digitizer.lvlib/3458A Digitizer Session.ctl" = cluster{"channels":T18[], "sync unit":T19, "awg unit":T21, "sync mode":T40, "streaming mode":bool, "idn mode":T41, "sampling mode":T42, "sample memory [B]":i32, "proc setup":T43, "sample size [B]":i32, "sample count":i32, "aux data":T45, "ranges [V]":dbl[], "aperture [s]":dbl, "LEVEL trigger":T46, "trigger mode":T47, "measure temp.?":bool, "disp mesages":string[], "shared bus?":bool, "disable display?":bool, "aper mode":T48, "aper rules":dbl[][], "multiplex":T49, "F8588 lpf":T50, "F8588 pll":T51, "F8588 couple":T52, "fs":T53, "fs mode":T55, "init timestamp":timestamp, "last report timestamp":timestamp}
  T18 = typedef "3458A Virtual Digitizer.lvlib/3458A Virtual Channel Config.ctl" = cluster{"VISA":refnum<visa-resource-name>, "Range [Vpk]":dbl, "btn clr":bool, "btn up":bool, "btn down":bool, "F8588":bool, "F8588 guard":bool}
  T19 = typedef "Counter.lvlib/Counter Session.ctl" = cluster{"VISA":refnum<visa-resource-name>, "type":T20}
  T20 = typedef "Counter.lvlib/Counter Type.ctl" = enum16{"Picotest U6200A", "dummy"}
  T21 = typedef "AWG.lvlib/AWG Session.ctl" = cluster{"type":T22, "VISA":refnum<visa-resource-name>, "enable 10MHz ref":bool, "cmi ckd2":T23, "cmi sync v3":T26, "trigger":T35, "HMF2500 cfg":T39}
  T22 = typedef "AWG.lvlib/AWG Type.ctl" = enum16{"Agilent 331xxA to 332xxA", "Agilent 335xxA to 336xxA", "Tektronix AFG3101C", "R&S HMF25xx", "CMI Clock Divider v2", "CMI Sync Unit V3", "dummy"}
  T23 = typedef "AWG.lvlib/CMI ckd2 Session.ctl" = cluster{"VISA":refnum<visa-resource-name>, "clock source":T24, "manual ref clk":bool, "ref clock [Hz]":dbl, "div mode":T25}
  T24 = typedef "AWG.lvlib/CMI ckd2 Source Mode.ctl" = enum16{"Auto", "LF clock", "HF clock", "Internal"}
  T25 = typedef "AWG.lvlib/CMI ckd2 Divisor Mode.ctl" = enum16{"Set divisor directly", "Set divisor by frequency"}
  T26 = typedef "AWG.lvlib/CMI Sync Unit V3.lvlib/CMI Sync V3 session.ctl" = cluster{"VISA":refnum<visa-resource-name>, "baud rate [bd/s]":i32, "source":T27, "hv range":T28, "fsrc is fixed":bool, "fsrc [Hz]":dbl, "freq integ [s]":dbl, "freq filter":i32, "trig level":T29, "chn1 mode":T30, "chn1 level":T31, "chn2 mode":T32, "chn2 level":T31, "chn2 div":i32, "chn3 mode":T33, "chn3 level":T31, "chn1 div entry":T34, "chn1 dev limit [%]":dbl, "chn1 check dev":bool}
  T27 = typedef "AWG.lvlib/CMI Sync Unit V3.lvlib/CMI Sync V3 Reference Clock Source.ctl" = enum16{"Auto", "Internal", "Logic", "Sine", "HV"}
  T28 = typedef "AWG.lvlib/CMI Sync Unit V3.lvlib/CMI Sync V3 HV input Range.ctl" = enum16{"10V", "60V", "250V", "1kV"}
  T29 = typedef "AWG.lvlib/CMI Sync Unit V3.lvlib/CMI Sync V3 Trigger Input Level.ctl" = enum16{"LVCMOS 3V3", "TTL 5V"}
  T30 = typedef "AWG.lvlib/CMI Sync Unit V3.lvlib/CMI Sync V3 Channel 1 Mode.ctl" = enum16{"Source divider", "DDS absolute", "DDS ratio", "DDS ratio M/N"}
  T31 = typedef "AWG.lvlib/CMI Sync Unit V3.lvlib/CMI Sync V3 Channel Output Levels.ctl" = enum16{"Positive 3V3", "Negative 3V3", "Positive 5V", "Negative 5V"}
  T32 = typedef "AWG.lvlib/CMI Sync Unit V3.lvlib/CMI Sync V3 Channel 2 Mode.ctl" = enum16{"Source divider", "Chn 1 divide"}
  T33 = typedef "AWG.lvlib/CMI Sync Unit V3.lvlib/CMI Sync V3 Channel 3 Mode.ctl" = enum16{"Chn 1 Active", "Chn 2 Active", "Chn 1 Trigger", "Chn 2 Trigger", "Gate", "PPS", "10MHz"}
  T34 = typedef "AWG.lvlib/CMI Sync Unit V3.lvlib/CMI Sync V3 Channel 1 Divisor Entry Mode.ctl" = enum16{"Set divisor directly", "Calculate nearest divisor from measured fx"}
  T35 = typedef "ADC Trig Config.ctl" = cluster{"source":T36, "slope":T37, "coupling":T38, "level [V]":dbl, "hysteresis [V]":dbl, "pre-trigger [%]":dbl}
  T36 = typedef "ADC Trig Mode Source.ctl" = enum16{"Immediate", "External", "Level"}
  T37 = typedef "ADC Trig Slope.ctl" = enum16{"POS", "NEG"}
  T38 = typedef "ADC Trig Coupling.ctl" = enum16{"DC", "AC"}
  T39 = typedef "AWG.lvlib/HMF2500 Config.ctl" = cluster{"Baud Rate":u32, "Parity":u16, "Data Bits":u16, "Flow Control":u16}
  T40 = typedef "3458A Virtual Digitizer.lvlib/3458A Sync Mode.ctl" = enum16{"MASTER-SLAVE, MASTER clocked by TIMER", "MASTER-SLAVE, MASTER clocked by AWG", "ALL clocked by AWG", "MASTER-SLAVE, ALL clocked by TIMER", "ALL clocked by AWG with DFLL"}
  T41 = typedef "3458A Virtual Digitizer.lvlib/3458A Idn Mode.ctl" = enum16{"Auto", "Sequential (chn A, chn B, ...)", "From calibration string"}
  T42 = typedef "3458A Virtual Digitizer.lvlib/3458A Digitizing Low Levels.lvlib/Sampling Mode.ctl" = enum16{"DCV", "DSDC", "DSAC"}
  T43 = typedef "3458A Virtual Digitizer.lvlib/3458A Digitizing Process Options.ctl" = cluster{"channel id":i32, "packet size [smpl]":i32, "current timeout [s]":dbl, "blk2blk timeout [s]":dbl, "event time":timestamp, "stop notifier":refnum<notifier>, "data queues":refnum<queue>[], "proc refs":refnum<vi>[], "bus semaphore":T44}
  T44 = typedef "Semaphore RefNum" = refnum<k1>
  T45 = typedef "3458A Virtual Digitizer.lvlib/3458A Aux Record Data.ctl" = cluster{"channel id":i32, "valid?":bool[], "gain [V]":dbl[], "timestamp [s]":dbl[], "Ts [s]":dbl, "abs timestamp":timestamp, "t [deg C]":dbl[], "multiplex timestamp [s]":dbl, "only multiplex?":bool, "multiplex smpl offset":i64, "overflow?":bool}
  T46 = typedef "3458A Virtual Digitizer.lvlib/3458A Digitizing Low Levels.lvlib/Level Setup.ctl" = cluster{"edge":enum16{"POS", "NEG"}, "level [V]":dbl, "coupling":enum16{"DC", "AC"}}
  T47 = typedef "3458A Virtual Digitizer.lvlib/3458A Digitizing Low Levels.lvlib/First Sample Trigger.ctl" = enum16{"AUTO", "EXT", "SYN", "SGL", "HOLD", "LEVEL"}
  T48 = typedef "3458A Virtual Digitizer.lvlib/3458A Aperture Selection Mode.ctl" = enum16{"Manual", "Maximum", "Table"}
  T49 = typedef "3458A Virtual Digitizer.lvlib/3458A Multiplexing Config.ctl" = cluster{"cycles":i32, "delay [s]":dbl, "enabled":bool, "overhead [s]":dbl, "tot smpls":i64, "sub-rec":i32, "overhead [%]":dbl, "emulated":bool}
  T50 = typedef "F8588A Low Pass Filter.ctl" = enum16{"Off", "100 kHz", "3 MHz"}
  T51 = typedef "F8588A Phase Lock.ctl" = enum16{"Off", "1 MHz", "10 MHz"}
  T52 = typedef "F8588A Coupling.ctl" = enum16{"AC, 1 MOhm", "AC, 10 MOhm", "DC, 1 MOhm", "DC, 10 MOhm", "DC, auto"}
  T53 = typedef "3458A Virtual Digitizer.lvlib/3458A Sampling Rate.ctl" = cluster{"freq mode":T54, "fs [Hz]":dbl, "fref [Hz]":dbl, "mul":dbl, "div":dbl}
  T54 = typedef "AWG.lvlib/AWG Clock Setup Mode.ctl" = enum16{"fs or Ts", "fs or Ts with fref", "fref/N", "fref*M/N", "fref*Ratio"}
  T55 = typedef "3458A Sample Rate Mode.ctl" = enum16{"fs or Ts", "fs*M/N"}
  T56 = typedef "DSDLL Virtual Digitizer.lvlib/DSDLL Session.ctl" = cluster{"dsdll":T57, "channels":i32, "device id":i32, "channel idns":string[], "proc setup":T59, "samples count":i32, "fs [Hz]":dbl}
  T57 = typedef "dsdll.lvlib/dsdll_instance.ctl" = cluster{"dsdll path":path, "dsdll handle":u8[], "output devices":T58[], "capture devices":T58[]}
  T58 = typedef "dsdll.lvlib/dsdll_device_record.ctl" = cluster{"guid":u8[], "name":string}
  T59 = typedef "DSDLL Virtual Digitizer.lvlib/DSDLL Process Config.ctl" = cluster{"packet size [smpl]":i32, "current timeout [s]":dbl, "blk2blk timeout [s]":dbl, "event time":timestamp, "data queue":refnum<queue>, "stop notifier":refnum<notifier>, "proc ref":refnum<vi>}
  T60 = typedef "ADC Type.ctl" = enum16{"niScope", "3458A", "DirectSound DLL", "Keysight DSO", "cDAQ ADC", "CMI ADS127L21", "dummy"}
  T61 = typedef "SimAdc Config.ctl" = cluster{"channels":T62[], "range [V]":dbl, "Ts step [s]":dbl, "time [s]":dbl, "fs [Hz]":dbl, "count":i64, "smpl offset":i64, "set count":i64, "bit res":i32}
  T62 = typedef "SimAdc Channel Cfg.ctl" = cluster{"harmonics":dbl[][], "btn clear":bool, "noise":dbl, "fundamental [Hz]":dbl}
  T63 = typedef "ADC On Close Action.ctl" = enum16{"Immediate reset", "Delayed reset"}
  T64 = typedef "MPX Session.ctl" = cluster{"Type":T65, "gen com ssn":T66, "delay before [s]":dbl, "delay post [s]":dbl, "sequence":string[], "enabled":bool, "ref timestamp [s]":dbl, "idn string":string, "dev niScope":refnum<k15>, "niScope idx":i32, "QPMX ssn":T70, "VISA mux ssn":T73}
  T65 = typedef "MPX Type.ctl" = enum16{"Dummy", "Generic - COM port", "Generic - niScope PFI", "Generic - VISA commands", "QPMX"}
  T66 = typedef "GCOMM Session.ctl" = cluster{"visa":refnum<visa-resource-name>, "primary":T67, "secondary":T67, "channels":T68[]}
  T67 = typedef "GCOMM Signal.ctl" = enum16{"None", "DTR", "RTS"}
  T68 = typedef "GCOMM Virtual Channel.ctl" = cluster{"Primary:":T69, "Secondary:":T69, "btn clr":bool, "btn up":bool, "btn down":bool, "Tag:":string}
  T69 = typedef "GCOMM Logic State.ctl" = enum16{"OFF", "ON"}
  T70 = typedef "QPMX Session.ctl" = cluster{"visa":refnum<visa-resource-name>, "switch mode":T71, "sequence":bool[][], "timing delays":u32[], "polarity":T72, "ss delay (s)":dbl, "internal timer (s)":dbl, "Last loaded sequence file":path, "startup delay (s)":dbl}
  T71 = typedef "QPMX switch mode.ctl" = enum16{"Switched by TWM", "Switched by external clock", "Switched by internal clock"}
  T72 = typedef "QPMX polarity.ctl" = enum16{"Positive", "Negative"}
  T73 = typedef "GVISA Mux Session.ctl" = cluster{"VISA":refnum<visa-resource-name>, "paths":T74[], "idn command":string, "serial cfg":T75}
  T74 = typedef "GVISA Mux Path Entry.ctl" = cluster{"Tag:":string, "Command:":string, "btn clr":bool, "btn up":bool, "btn down":bool}
  T75 = typedef "met_serial_setup.ctl" = cluster{"Baud rate":i32, "Data bits":i32, "Parity":i32, "Stop bits":i32, "Flow control":i32, "End Mode Read":enum16{"None", "Last Bit", "TermChar"}, "End Mode Write":enum16{"None", "Last Bit", "TermChar"}, "Term character":u8, "Term enable":bool}
  T76 = typedef "KeDSO session.ctl" = cluster{"VISA":refnum<visa-resource-name>, "channels":T77[], "bw limit [Hz]":dbl, "resolution":T78, "trig noise reject":enum16{"Normal", "High Sensitivity"}, "N":i64, "trigger config":T79, "fs [Hz]":dbl, "timeout stop":timestamp, "waiting for opc":bool, "fetch offset [smpl]":i64, "abs timestamp":timestamp, "ranges [V]":dbl[], "decimation":dbl, "ext ref":bool, "emulate aperture":bool, "model":T81}
  T77 = typedef "KeDSO Virtual Channel.ctl" = cluster{"Channel":i32, "Range [Vpk]":dbl, "btn clr":bool, "btn up":bool, "btn down":bool, "Offset [V]":dbl, "Coupling":enum16{"DC", "DC50", "AC", "LFR1"}, "bw limit enab":bool}
  T78 = typedef "KeDSO High Resolution Mode.ctl" = enum16{"Basic", "High-res AUTO", "Min. 9-bits", "Min. 10-bits", "Min. 11-bits", "Min. 12-bits", "Fixed 11-bits", "Fixed 12-bits", "Fixed 13-bits", "Fixed 14-bits", "Fixed 15-bits", "Fixed 16-bits"}
  T79 = typedef "KeDSO Trigger Setup.ctl" = cluster{"trigger source":T80, "trigger slope":enum16{"Negative", "Positive", "Either"}, "level [V]":dbl, "hysteresis [V]":dbl, "pre-trig [%]":i32}
  T80 = typedef "KeDSO Trigger Source.ctl" = enum16{"Immediate", "Level", "AUX"}
  T81 = typedef "Agilent 90000 Series.lvlib/DSO type.ctl" = enum16{"DSO91304", "DSO91204", "DSO90804", "DSO90604", "DSO90404", "DSO90254", "DSA91304", "DSA91204", "DSA90804", "DSA90604", "DSA90404", "DSA90254", "DSO9104", "DSO9254", "DSO9404", "MSO9104", "MSO9254", "MSO9404", "MSO9064", "DSO9064", "DSOX91604", "DSOX92004", "DSOX92504", "DSOX92804", "DSOX93204", "DSO93004", "DSO9024H", "DSO9054H", "DSO9104H", "DSO9204H", "DSOS054A", "DSOS104A", "DSOS204A", "DSOS254A", "DSOS404A", "DSOS604A", "DSOS804A", "MSOS054A", "MSOS104A", "MSOS204A", "MSOS254A", "MSOS404A", "MSOS604A", "MSOS804A", "DSAX96204Q", "DSOX96204Q", "DSAX95004Q", "DSOX95004Q", "DSAX93304Q", "DSOX93304Q", "DSAX92504Q", "DSOX92504Q", "DSAX92004Q", "DSOX92004Q"}
  T82 = typedef "cDAQ Session.ctl" = cluster{"mclk [Hz]":dbl, "ADC task":refnum<k21>, "mclk reference":string, "fs [Hz]":dbl, "queue adc cmd":refnum<queue>, "queue adc data":refnum<queue>, "adc proc ref":refnum<vi>, "channels":T83[], "last channels":T83[], "timeout":timestamp, "N":i32, "mclk mode":T84, "ext mclk source":tag}
  T83 = typedef "cDAQ Virtual Channel.ctl" = cluster{"Device":tag, "Channel id":i32, "btn clr":bool, "btn up":bool, "btn down":bool}
  T84 = typedef "cDAQ Master Clock Mode.ctl" = enum16{"Free running", "Export master clock", "Import master clock"}
  T85 = typedef "CMI ADS127L21 - Session.ctl" = cluster{"VISA":refnum<visa-resource-name>, "chn list":i32[], "record size":i32, "phys. channels":i32, "adc fifo size":i32, "channels":T86[], "ext refclk?":bool, "fs [Hz]":dbl, "ext refclk [Hz]":dbl, "meas refclk [Hz]":dbl, "EXTOUT mode":T90, "EXTOUT polarity":T91, "EXTOUT divisor":i32}
  T86 = typedef "CMI ADS127L21 - Record Channel.ctl" = cluster{"Range [Vpk]":T87, "Channel":i32, "Mode":T88, "Impedance":T89, "btn clr":bool, "btn up":bool, "btn down":bool}
  T87 = typedef "CMI ADS127L21 - Input Range.ctl" = dbl
  T88 = typedef "CMI ADS127L21 - Input Mode.ctl" = enum16{"Normal", "Inverted", "GND"}
  T89 = typedef "CMI ADS127L21 - Input Impedance.ctl" = enum16{"1M", "1k5"}
  T90 = typedef "CMI ADS127L21 - EXTOUT Mode.ctl" = enum16{"ADCCLK", "REFCLK", "SMPLCLK", "FIRST"}
  T91 = typedef "CMI ADS127L21 - EXTOUT Polarity.ctl" = enum16{"NORM", "INV"}
  T92 = typedef "Meas Sequence Item.ctl" = cluster{"config":T93, "data file path":path, "header file path":path, "group id":i32, "rec id":i32, "group done?":bool, "adc modified?":bool, "source modified?":bool, "progress [%]":dbl, "groups cnt":i32, "rec cnt":i32, "data file relative path":string, "meas root path":path, "calculate?":bool, "comment":string, "avg cnt":i32}
  T93 = typedef "Meas Sampling Configuration.ctl" = cluster{"count [smpl]":i64, "aperture [s]":dbl, "trigger":T35, "ranges [Vpk]":dbl[], "QWTB parameters":T94[], "sampling rate":T53}
  T94 = typedef "Meas Proc QWTB Algorithm Parameter Data.ctl" = cluster{"name":string, "numerics":dbl[], "strings":string[]}
  T95 = typedef "Meas Sequence Configuration.ctl" = cluster{"group setups":T93[], "rec count":i32, "range mode":T96, "fs mode":T97, "rng even":dbl, "rng odd":dbl, "folder":path, "name base":string, "meas id":i32, "settle [s]":dbl, "comment":string, "avg count":i32, "fs-abs-fr fr":dbl, "fs-abs-fr fs":dbl, "fs-div fr":dbl, "fs-div div":dbl, "fs-mn fr":dbl, "fs-mn mul":dbl, "fs-mn div":dbl, "fs-rat fr":dbl, "fs-rat rat":dbl}
  T96 = typedef "Meas Range Mode.ctl" = enum16{"Keep defaults", "Set All channels", "Set Odd and Even channels"}
  T97 = typedef "Meas Sampling Rate Mode.ctl" = enum16{"Frequency", "Period"}
  T98 = typedef "GOLPI Multi Process.lvlib/golpi_session_ref.ctl" = refnum<vi>
  T99 = typedef "Meas Process Config.ctl" = cluster{"mode":T100, "call after avgs?":bool, "calculate?":bool, "raw mode":T101, "QWTB":T103}
  T100 = typedef "Meas Process Mode.ctl" = enum16{"Raw", "QWTB"}
  T101 = typedef "Meas Process Raw Config.ctl" = cluster{"command":string, "result mode":T102, "res variable":string}
  T102 = typedef "Meas Process Raw Result Mode.ctl" = enum16{"Display console output (only Octave)", "Display string variable", "Display result file %respath%"}
  T103 = typedef "Meas Proc QWTB Setup.ctl" = cluster{"QWTB path":path, "alg filter path":string, "alg ids":string[], "alg parameters":string[], "parsed parameters":T94[], "selected alg id":string, "selected unc mode":T104, "qwtb mcc":i32, "qwtb timeout":i32, "qwtb covg":dbl, "qwtb ofs":i64, "qwtb lim data":i64, "multicore":T105, "unc once?":bool, "qwtb tstemp":T107, "octave reset":bool, "exec mode":T108}
  T104 = typedef "Meas Proc QWTB Uncertainty Mode.ctl" = enum16{"None", "GUF", "Monte Carlo"}
  T105 = typedef "Meas Proc QWTB Multicore Setup.ctl" = cluster{"jobs folder":path, "cores":i32, "max jobs":i32, "mode":T106}
  T106 = typedef "Meas Proc QWTB Multicore Type.ctl" = enum16{"Singlecore", "Multicore", "Multistation"}
  T107 = typedef "Meas Process Time Stamp Mode.ctl" = enum16{"Enabled (default)", "Disabled", "Relative to 1. record"}
  T108 = typedef "Meas Proc QWTB Exec Mode.ctl" = enum16{"Single-core", "Parallel Record Processing"}
  T109 = typedef "Corr Setup.ctl" = cluster{"transducers":cluster{"channels":T110[], "last path":path, "root path":path}, "digitizer":T111}
  T110 = typedef "Corr Tranducer Item.ctl" = cluster{"Path":path, "Ratio:":string, "Name:":string, "btn rem":bool, "btn up":bool, "btn down":bool, "s.n.:":string, "btn open":bool, "ratio o/i":dbl, "chn hi":u16, "chn lo":u16, "Phase index":i32, "btn edit":bool, "mpx chn":u16, "btn vdx1":bool, "btn csx1":bool, "invert":bool}
  T111 = typedef "Corr Digitizers.ctl" = cluster{"last path":path, "channel paths":path[], "channel idns":string[], "correction name":string, "channel names":string[], "folders to copy":path[], "channel valid":bool[], "correction path":path, "correction rel path":string, "rel folders to copy":string[], "root path":path}
  T112 = typedef "Assist Panel Setup.ctl" = cluster{"P":i32, "Q":i32, "rel shift":dbl, "ref freq":dbl, "min fs":dbl, "max fs tol":dbl, "min int":dbl, "max int":dbl, "max err":dbl, "max timeout":dbl}
  T113 = typedef "varilib.lvlib/SGUI Assign References Mode.ctl" = enum16{"Add to stack", "Overwrite", "Release last", "Release ID"}
  T114 = typedef "Parameter Matrix Operation.vi" = enum16{"Initialize", "On Row Select", "On Menu Drop", "On Menu Select", "Get values"}
  T115 = typedef "Meas Proc QWTB Algorithm Flags.ctl" = cluster{"supports multiple records?":bool, "supports differential transducer?":bool, "dual input algorithm?":bool, "has GUF?":bool, "has MCM?":bool}
  T116 = typedef "LVPoint32TypeDef.ctl" = cluster{"Horizontal":i32, "Vertical":i32}
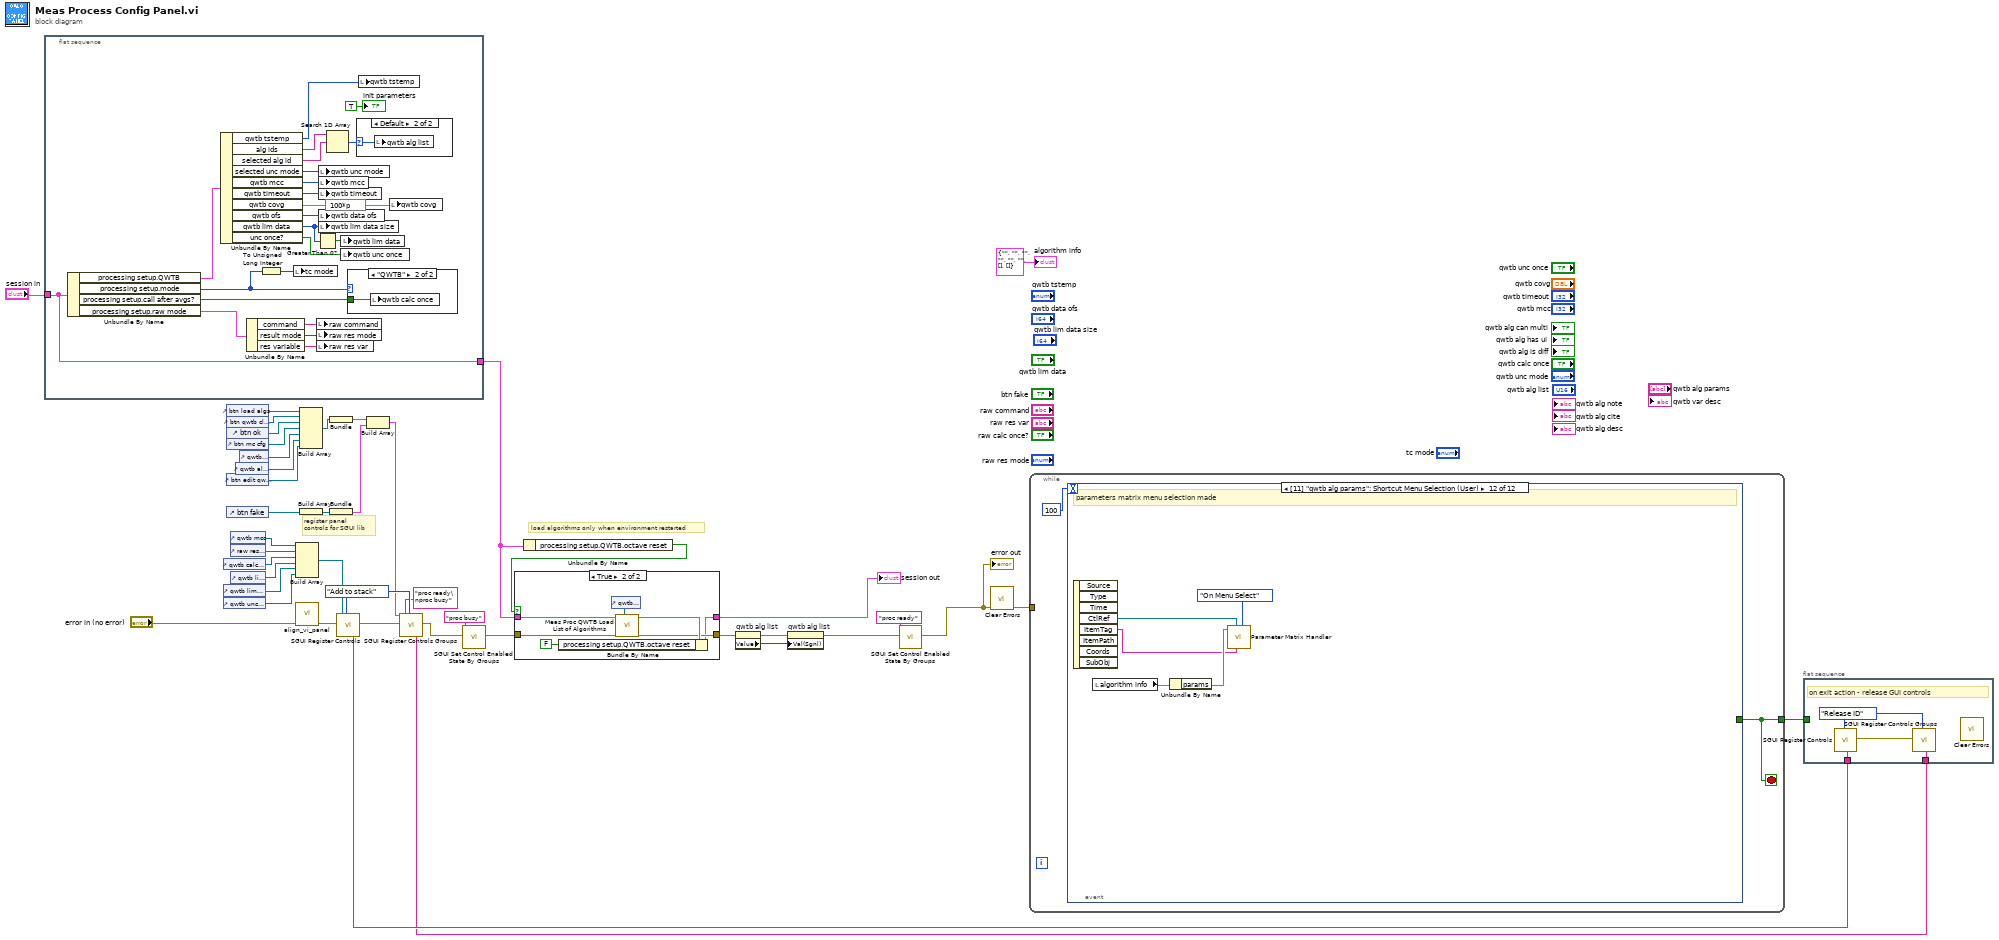
[diagram p0: block diagram]
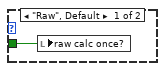
[diagram p4: hidden frame]
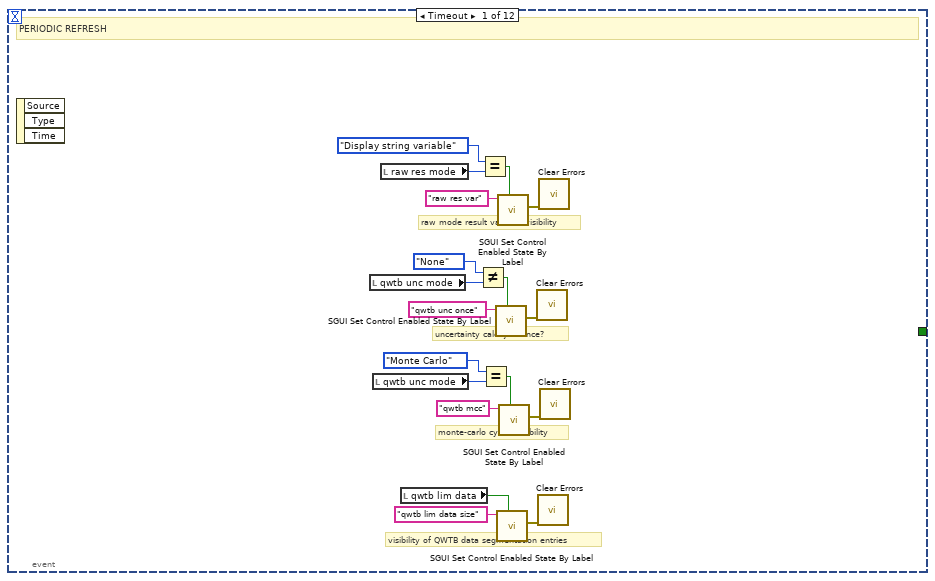
[diagram p5: hidden frame]
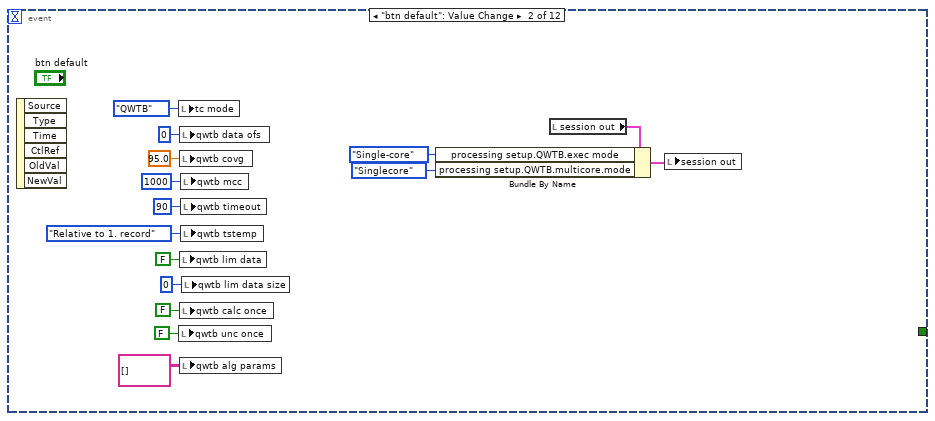
[diagram p6: hidden frame]
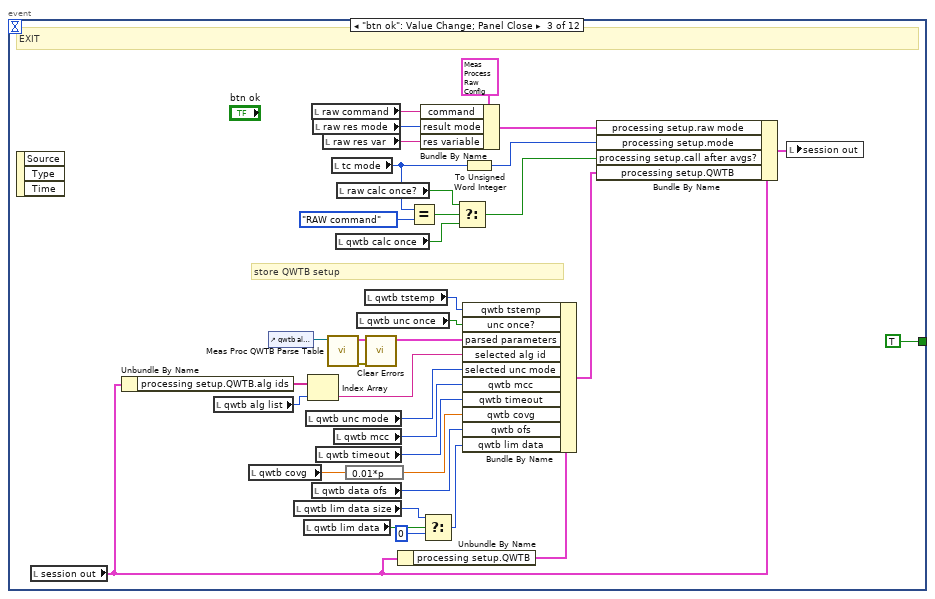
[diagram p7: hidden frame]
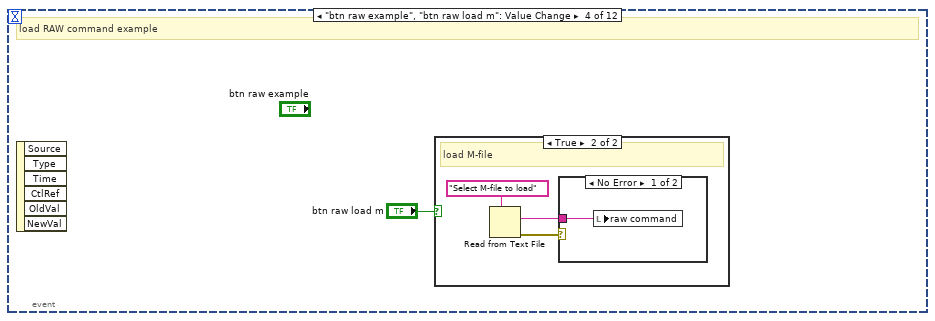
[diagram p8: hidden frame]
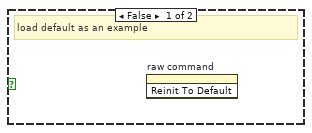
[diagram p9: hidden frame]
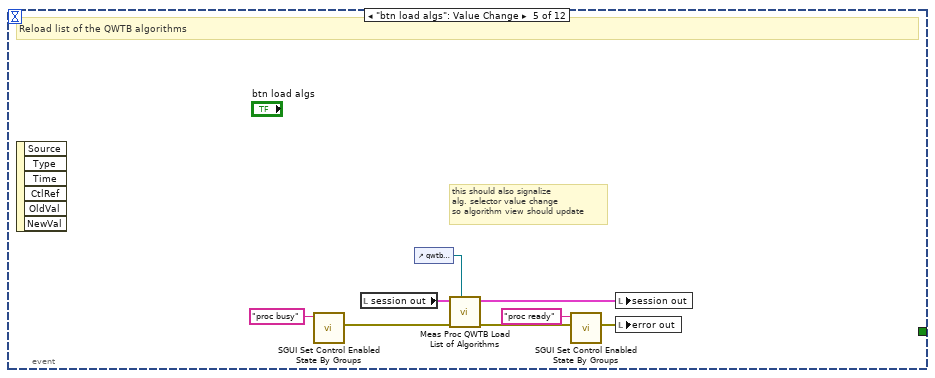
[diagram p11: hidden frame]
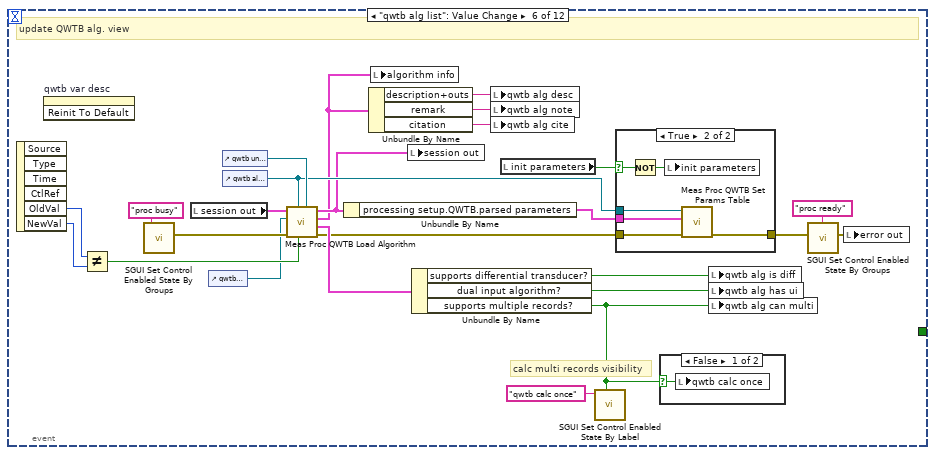
[diagram p12: hidden frame]
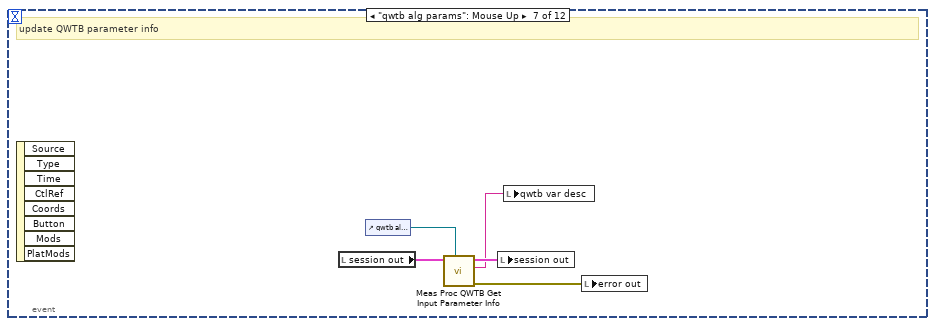
[diagram p15: hidden frame]
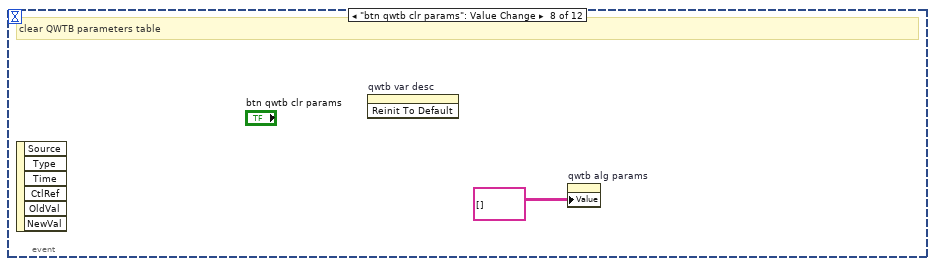
[diagram p16: hidden frame]
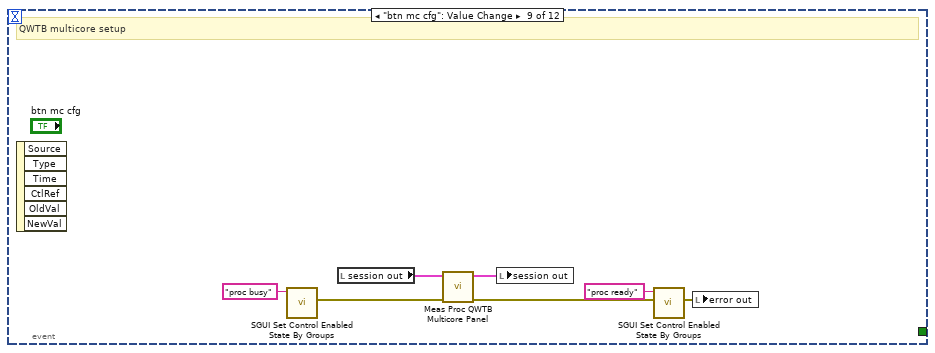
[diagram p17: hidden frame]
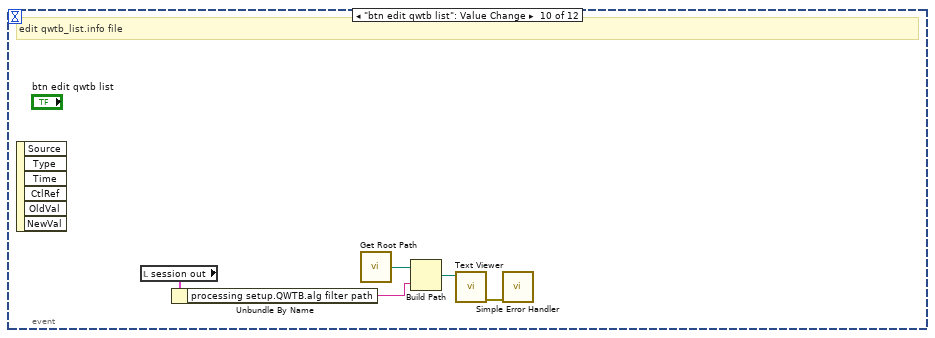
[diagram p18: hidden frame]
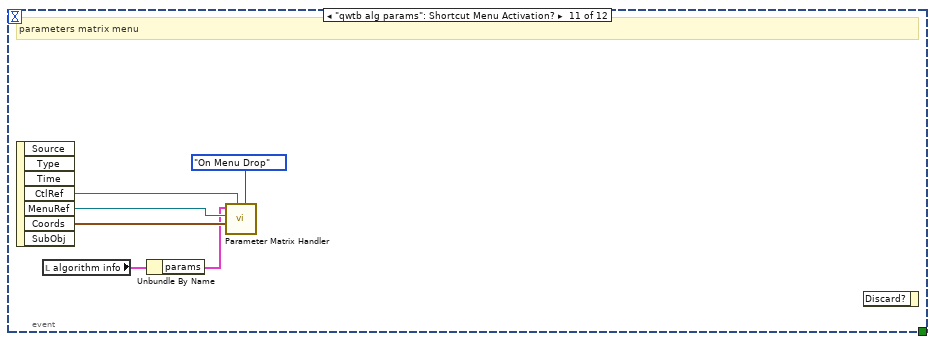
[diagram p19: hidden frame]
diagram:
  w32 = SGUI_Assign_References_Mode."Add to stack" ("register mode (overwrite)")
  # "load algorithms only when environment restarted"
  # "register panel\ncontrols for SGUI lib"
  n1 = flat-sequence {
    tunnel: "session in" -> [w57]
    tunnel: [w57] -> w8
    frame #0 {
      n2 = Unbundle By Name(w57) -> ("processing setup.QWTB"=w59:T103, "processing setup.mode"=w61:T100, "processing setup.call after avgs?"=w60:bool, "processing setup.raw mode"=w65:T101)
      n3 = Unbundle By Name(w59) -> ("qwtb tstemp"=w44:T107, "alg ids"=w52:string[], "selected alg id"=w51:string, "selected unc mode"=w58:T104, "qwtb mcc"=w56:i32, "qwtb timeout"=w55:i32, "qwtb covg"=w54:dbl, "qwtb ofs"=w48:i64, "qwtb lim data"=w46:i64, "unc once?"=w45:bool)
      n4 = Unbundle By Name(w65) -> ("command"=w64:string, "result mode"=w63:T102, "res variable"=w62:string)
      n5 = To Unsigned Long Integer(number=w61) -> (unsigned 32bit integer=w66:u32)
      n6 = local write "tc mode"(w66) -> ()
      n7 = Greater Than 0?(x=w46) -> (x > 0?=w47:bool)
      n8 = local write "raw command"(w64) -> ()
      n9 = local write "raw res mode"(w63) -> ()
      n10 = local write "raw res var"(w62) -> ()
      n11 = local write "qwtb unc mode"(w58) -> ()
      n12 = local write "qwtb mcc"(w56) -> ()
      n13 = local write "qwtb timeout"(w55) -> ()
      n14 = local write "qwtb data ofs"(w48) -> ()
      n15 = local write "qwtb lim data size"(w46) -> ()
      n16 = expression code="100*p"(w54) -> (w53:dbl)
      n17 = Search 1D Array(1D array=w52, element=w51) -> (index of element=w50:i32)  [unwired: 1 in]
      n18 = local write "qwtb lim data"(w47) -> ()
      n19 = local write "qwtb unc once"(w45) -> ()
      n20 = case shown="\"QWTB\"" w61 {
        tunnel: w60 -> [w68 w69]
        frame "Raw", Default {
          n21 = local write "raw calc once?"(w68) -> ()
        }
        frame "QWTB" {
          n22 = local write "qwtb calc once"(w69) -> ()
        }
      }
      n23 = case shown="Default" w50 {
        selector: w50 -> [_ w67]
        frame -1 {
        }
        frame Default {
          n24 = local write "qwtb alg list"(w67) -> ()
        }
      }
      n25 = local write "qwtb tstemp"(w44) -> ()
      n26 = local write "qwtb covg"(w53) -> ()
      "init parameters" <- TRUE ("init parameters")
    }
  }
  n27 = control-ref of="qwtb calc once"() -> (w36:refnum<vi>)
  n28 = control-ref of="qwtb lim data"() -> (w13:refnum<vi>)
  n29 = control-ref of="qwtb unc once"() -> (w11:refnum<vi>)
  n30 = control-ref of="btn load algs"() -> (w24:refnum<vi>)
  n31 = control-ref of="btn qwtb clr params"() -> (w23:refnum<vi>)
  n32 = control-ref of="btn ok"() -> (w22:refnum<vi>)
  n33 = control-ref of="btn mc cfg"() -> (w12:refnum<vi>)
  n34 = control-ref of="btn fake"() -> (w21:refnum<vi>)
  n35 = control-ref of="btn edit qwtb list"() -> (w2:refnum<vi>)
  n36 = control-ref of="qwtb mcc"() -> (w35:refnum<vi>)
  n37 = control-ref of="raw res var"() -> (w42:refnum<vi>)
  n38 = control-ref of="qwtb lim data size"() -> (w14:refnum<vi>)
  n39 = control-ref of="qwtb alg params"() -> (w9:refnum<vi>)
  n40 = control-ref of="qwtb alg list"() -> (w10:refnum<vi>)
  n41 = Build Array(w35, w42, w36, w14, w13, w11) -> (w43:refnum<vi>[])
  n42 = call "align_vi_panel.vi"("error in"="error in (no error)") -> ("error out"=w39:errorcluster)  [unwired: 10 in]
  n43 = Build Array(w24, w23, w22, w12, w10, w9, w2) -> (w30:refnum<vi>[])
  n44 = Build Array(w21) -> (w28:refnum<vi>[])
  n45 = Bundle(w30) -> (w31:cluster{refnum<vi>[]})  [unwired: 1 in]
  n46 = Bundle(w28) -> (w29:cluster{refnum<vi>[]})  [unwired: 1 in]
  n47 = call "SGUI Register Controls.vi"("error in"=w39, "control references (empty)"=w43, "register mode (overwrite)"=w32) -> ("assigned ID"=w34:string, "error out"=w33:errorcluster)  [unwired: 14 in, 1 out]
  n48 = Build Array(w31, w29) -> (w26:cluster{refnum<vi>[]}[])
  n49 = call "SGUI Register Controls Groups.vi"("control groups"=w26, "error in"=w33, "groups names"="proc ready\nproc busy", "register mode (overwrite)"=w32) -> ("assigned ID"=w25:string, "error out"=w17:errorcluster)  [unwired: 14 in]
  n50 = call "SGUI Set Control Enabled State By Groups.vi"("error in"=w17, "group name to enable (none)"="proc busy") -> ("error out"=w18:errorcluster)  [unwired: 8 in, 1 out]
  n51 = Unbundle By Name(w8) -> ("processing setup.QWTB.octave reset"=w7:bool)
  n52 = case shown="True" w7 {
    tunnel: [w71 w73] -> w37
    tunnel: w8 -> [w71 w76]
    tunnel: w18 -> [w70 w75]
    tunnel: [w70 w74] -> w6
    frame False {
    }
    frame True {
      n53 = control-ref of="qwtb alg list"() -> (w77:refnum<vi>)
      n54 = call "Meas Proc QWTB Load List of Algorithms.vi"("menu ring ref"=w77, "error in"=w75, "session in"=w76) -> ("error out"=w74:errorcluster, "session out"=w78:T4)  [unwired: 6 in, 1 out]
      n55 = Bundle By Name(cluster=w78, "processing setup.QWTB.octave reset"=FALSE) -> (w73:T4)
    }
  }
  "session out" <- w37
  n56 = property on="qwtb alg list" class="Ring (strict)"(error in=w6) -> (error out=w5:errorcluster, "Value"=w4:u16)  [unwired: 1 in, 1 out]
  n57 = property on="qwtb alg list" class="Ring (strict)"(error in=w5, "Val(Sgnl)"=w4) -> (error out=w3:errorcluster)  [unwired: 1 in, 1 out]
  n58 = call "SGUI Set Control Enabled State By Groups.vi"("error in"=w3, "group name to enable (none)"="proc ready") -> ("error out"=w15:errorcluster)  [unwired: 8 in, 1 out]
  "error out" <- w15
  n59 = call <vilib>:"Clear Errors.vi"("error in (no error)"=w15) -> ("error out"=w41:errorcluster)  [unwired: 5 in, 1 out]
  n60 = while {
    tunnel: w41 -> [_]
    tunnel: [w79] -> w40
    stop <- w79 stop-if-true
    n61 = event shown="[11] \"qwtb alg params\": Shortcut Menu Selection (User)" {
      selector: _ -> [_ _ _ _ _ _ _ _ _ _ _ _]
      dyn-events: _ -> [_ _ _ _ _ _ _ _ _ _ _ _]
      timeout: 100 -> [_ _ _ _ _ _ _ _ _ _ _ _]
      tunnel: [_ _ TRUE _ _ _ _ _ _ _ _ _] -> w79
      event Timeout {
        # "uncertainty calc. just once?"
        # "visibility of QWTB data segmentation entries"
        # "monte-carlo cycles visibility"
        # "raw mode result variable visibility"
        # "PERIODIC REFRESH"
        n62 = event-data() -> ()  [unwired: 1 in, 3 out]
        n63 = local read "qwtb unc mode"() -> (w84:T104)
        n64 = local read "qwtb unc mode"() -> (w90:T104)
        n65 = local read "raw res mode"() -> (w98:T102)
        n66 = local read "qwtb lim data"() -> (w88:bool)
        n67 = Not Equal?(x=Meas_Proc_QWTB_Uncertainty_Mode."None", y=w84) -> (x != y?=w83:bool)
        n68 = Equal?(x=Meas_Process_Raw_Result_Mode."Display string variable", y=w98) -> (x = y?=w96:bool)
        n69 = Equal?(x=Meas_Proc_QWTB_Uncertainty_Mode."Monte Carlo", y=w90) -> (x = y?=w91:bool)
        n70 = call "SGUI Set Control Enabled State By Label.vi"("labels (empty)"="qwtb unc once", "Enabled? (False)"=w83) -> ("error out"=w81:errorcluster)  [unwired: 8 in, 1 out]
        n71 = call "SGUI Set Control Enabled State By Label.vi"("labels (empty)"="qwtb lim data size", "Enabled? (False)"=w88) -> ("error out"=w86:errorcluster)  [unwired: 8 in, 1 out]
        n72 = call "SGUI Set Control Enabled State By Label.vi"("labels (empty)"="raw res var", "Enabled? (False)"=w96) -> ("error out"=w94:errorcluster)  [unwired: 8 in, 1 out]
        n73 = call "SGUI Set Control Enabled State By Label.vi"("labels (empty)"="qwtb mcc", "Enabled? (False)"=w91) -> ("error out"=w93:errorcluster)  [unwired: 8 in, 1 out]
        n74 = call <vilib>:"Clear Errors.vi"("error in (no error)"=w81) -> ()  [unwired: 5 in, 2 out]
        n75 = call <vilib>:"Clear Errors.vi"("error in (no error)"=w86) -> ()  [unwired: 5 in, 2 out]
        n76 = call <vilib>:"Clear Errors.vi"("error in (no error)"=w94) -> ()  [unwired: 5 in, 2 out]
        n77 = call <vilib>:"Clear Errors.vi"("error in (no error)"=w93) -> ()  [unwired: 5 in, 2 out]
      }
      event "btn default": Value Change {
        n78 = event-data() -> ()  [unwired: 1 in, 6 out]
        n79 = local write "tc mode"(enum32{"RAW command", "QWTB"}."QWTB" ("tc mode")) -> ()
        n80 = local write "qwtb unc once"(FALSE ("qwtb unc once")) -> ()
        n81 = local write "qwtb data ofs"(i64 0 ("qwtb data ofs")) -> ()
        n82 = local write "qwtb covg"(95.0 ("qwtb covg")) -> ()
        n83 = local write "qwtb lim data"(FALSE ("qwtb lim data")) -> ()
        n84 = local write "qwtb calc once"(FALSE ("qwtb calc once")) -> ()
        n85 = local write "qwtb alg params"(string[][] [] ("qwtb alg params")) -> ()
        n86 = local write "qwtb mcc"(1000 ("qwtb mcc")) -> ()
        n87 = local write "qwtb timeout"(90 ("qwtb timeout")) -> ()
        n88 = local write "qwtb tstemp"(Meas_Process_Time_Stamp_Mode."Relative to 1. record" ("qwtb tstemp")) -> ()
        n89 = local write "qwtb lim data size"(i64 0 ("qwtb lim data size")) -> ()
        n90 = local read "session out"() -> (w102:T4)
        n91 = Bundle By Name(cluster=w102, "processing setup.QWTB.exec mode"=Meas_Proc_QWTB_Exec_Mode."Single-core", "processing setup.QWTB.multicore.mode"=Meas_Proc_QWTB_Multicore_Type."Singlecore") -> (w99:T4)
        n92 = local write "session out"(w99) -> ()
      }
      event "btn ok": Value Change; Panel Close {
        # "store QWTB setup"
        # "EXIT"
        n93 = event-data() -> ()  [unwired: 1 in, 3 out]
        n94 = local read "session out"() -> (w124:T4)
        n95 = Unbundle By Name(w124) -> ("processing setup.QWTB.alg ids"=w123:string[])
        n96 = local read "qwtb alg list"() -> (w122:u16)
        n97 = local read "qwtb covg"() -> (w126:dbl)
        n98 = control-ref of="qwtb alg params"() -> (w134:refnum<vi>)
        n99 = local read "qwtb lim data size"() -> (w117:i64)
        n100 = local read "qwtb lim data"() -> (w119:bool)
        n101 = local read "qwtb unc mode"() -> (w132:T104)
        n102 = Index Array(array=w123, index=w122) -> (element=w121:string)
        n103 = local read "raw command"() -> (w147:string)
        n104 = local read "qwtb data ofs"() -> (w120:i64)
        n105 = local read "raw res mode"() -> (w146:T102)
        n106 = local read "qwtb timeout"() -> (w127:i32)
        n107 = local read "raw res var"() -> (w145:string)
        n108 = call "Meas Proc QWTB Parse Table.vi"("param table ref"=w134) -> ("error out"=w133:errorcluster, "qwtb parameters"=w135:T94[])  [unwired: 9 in]
        n109 = local read "tc mode"() -> (w137:enum32{"RAW command", "QWTB"})
        n110 = local read "qwtb mcc"() -> (w128:i32)
        n111 = local read "qwtb calc once"() -> (w130:bool)
        n112 = local read "raw calc once?"() -> (w141:bool)
        n113 = expression code="0.01*p"(w126) -> (w125:dbl)
        n114 = local read "qwtb unc once"() -> (w115:bool)
        n115 = local read "qwtb tstemp"() -> (w114:T107)
        n116 = call <vilib>:"Clear Errors.vi"("error in (no error)"=w133) -> ()  [unwired: 5 in, 2 out]
        n117 = Unbundle By Name(w124) -> ("processing setup.QWTB"=w129:T103)
        n118 = Equal?(x=w137, y=enum32{"RAW command", "QWTB"}."RAW command") -> (x = y?=w142:bool)
        n119 = Bundle By Name(cluster=T101 {"command"="", "result mode"=enum."Display result file %respath%", "res variable"=""} ("raw mode"), "command"=w147, "result mode"=w146, "res variable"=w145) -> (w144:T101)
        n120 = Select(t=w117, s=w119, f=i64 0) -> (s? t:f=w118:i64)
        n121 = Select(t=w141, s=w142, f=w130) -> (s? t:f=w140:bool)
        n122 = Bundle By Name(cluster=w129, "qwtb tstemp"=w114, "unc once?"=w115, "parsed parameters"=w135, "selected alg id"=w121, "selected unc mode"=w132, "qwtb mcc"=w128, "qwtb timeout"=w127, "qwtb covg"=w125, "qwtb ofs"=w120, "qwtb lim data"=w118) -> (w131:T103)
        n123 = To Unsigned Word Integer(number=w137) -> (unsigned 16bit integer=w136:u16)
        n124 = Bundle By Name(cluster=w124, "processing setup.raw mode"=w144, "processing setup.mode"=w136, "processing setup.call after avgs?"=w140, "processing setup.QWTB"=w131) -> (w139:T4)
        n125 = local write "session out"(w139) -> ()
      }
      event "btn raw example", "btn raw load m": Value Change {
        # "load RAW command example"
        n126 = event-data() -> ()  [unwired: 1 in, 6 out]
        n127 = case shown="True" "btn raw load m" {
          frame False {
            # "load default as an example"
            n128 = invoke on="raw command" class="Str" method="Reinit To Default"() -> ()  [unwired: 3 in, 3 out]
          }
          frame True {
            # "load M-file"
            n129 = Read from Text File(prompt (Open existing file)="Select M-file to load") -> (text=w150:string, error out=w151:errorcluster)  [unwired: 3 in, 2 out]
            n130 = case shown="No Error" w151 {
              tunnel: w150 -> [w153 _]
              frame No Error {
                n131 = local write "raw command"(w153) -> ()
              }
              frame Error {
              }
            }
          }
        }
      }
      event "btn load algs": Value Change {
        # "this should also signalize\nalg. selector value change\nso algorithm view should update"
        # "Reload list of the QWTB algorithms"
        n132 = event-data() -> ()  [unwired: 1 in, 6 out]
        n133 = call "SGUI Set Control Enabled State By Groups.vi"("group name to enable (none)"="proc busy") -> ("error out"=w158:errorcluster)  [unwired: 9 in, 1 out]
        n134 = local read "session out"() -> (w160:T4)
        n135 = control-ref of="qwtb alg list"() -> (w161:refnum<vi>)
        n136 = call "Meas Proc QWTB Load List of Algorithms.vi"("menu ring ref"=w161, "error in"=w158, "session in"=w160) -> ("error out"=w156:errorcluster, "session out"=w159:T4)  [unwired: 6 in, 1 out]
        n137 = call "SGUI Set Control Enabled State By Groups.vi"("error in"=w156, "group name to enable (none)"="proc ready") -> ("error out"=w155:errorcluster)  [unwired: 8 in, 1 out]
        n138 = local write "session out"(w159) -> ()
        n139 = local write "error out"(w155) -> ()
      }
      event "qwtb alg list": Value Change {
        # "calc multi records visibility"
        # "update QWTB alg. view"
        n140 = event-data() -> ("OldVal"=w167:u16, "NewVal"=w166:u16)  [unwired: 1 in, 4 out]
        n141 = invoke on="qwtb var desc" class="Str" method="Reinit To Default"() -> ()  [unwired: 3 in, 3 out]
        n142 = Not Equal?(x=w167, y=w166) -> (x != y?=w165:bool)
        n143 = call "SGUI Set Control Enabled State By Groups.vi"("group name to enable (none)"="proc busy") -> ("error out"=w177:errorcluster)  [unwired: 9 in, 1 out]
        n144 = local read "session out"() -> (w186:T4)
        n145 = control-ref of="qwtb alg list"() -> (w164:refnum<vi>)
        n146 = control-ref of="qwtb unc mode"() -> (w172:refnum<vi>)
        n147 = control-ref of="qwtb alg params"() -> (w171:refnum<vi>)
        n148 = call "Meas Proc QWTB Load Algorithm.vi"("qwtb unc mode ref"=w172, "alg. selection changed?"=w165, "param table ref"=w171, "error in"=w177, "qwtb alg selector"=w164, "session in"=w186) -> ("error out"=w174:errorcluster, "qwtb alg flags"=w182:T115, "algorithm info"=w162:T1, "session out"=w170:T4)  [unwired: 1 in, 1 out]
        n149 = Unbundle By Name(w170) -> ("processing setup.QWTB.parsed parameters"=w169:T94[])
        n150 = Unbundle By Name(w162) -> ("description+outs"=w184:string, "remark"=w185:string, "citation"=w183:string)
        n151 = local write "algorithm info"(w162) -> ()
        n152 = local write "session out"(w170) -> ()
        n153 = Unbundle By Name(w182) -> ("supports differential transducer?"=w181:bool, "dual input algorithm?"=w180:bool, "supports multiple records?"=w163:bool)
        n154 = local write "qwtb alg desc"(w184) -> ()
        n155 = local write "qwtb alg note"(w185) -> ()
        n156 = local write "qwtb alg cite"(w183) -> ()
        n157 = local read "init parameters"() -> (w168:bool)
        n158 = call "SGUI Set Control Enabled State By Label.vi"("labels (empty)"="qwtb calc once", "Enabled? (False)"=w163) -> ()  [unwired: 8 in, 2 out]
        n159 = case shown="True" w168 {
          selector: w168 -> [_ w190]
          tunnel: w174 -> [w188 w194]
          tunnel: [w188 w193] -> w173
          tunnel: w171 -> [_ w192]
          tunnel: w169 -> [_ w191]
          frame False {
          }
          frame True {
            n160 = Not(x=w190) -> (.not. x?=w189:bool)
            n161 = local write "init parameters"(w189) -> ()
            n162 = call "Meas Proc QWTB Set Params Table.vi"("error in"=w194, "qwtb parameters"=w191, "param table ref"=w192) -> ("error out"=w193:errorcluster)  [unwired: 8 in]
          }
        }
        n163 = case shown="False" w163 {
          selector: w163 -> [w187 _]
          frame False {
            n164 = local write "qwtb calc once"(w187) -> ()
          }
          frame True {
          }
        }
        n165 = local write "qwtb alg is diff"(w181) -> ()
        n166 = local write "qwtb alg has ui"(w180) -> ()
        n167 = local write "qwtb alg can multi"(w163) -> ()
        n168 = call "SGUI Set Control Enabled State By Groups.vi"("error in"=w173, "group name to enable (none)"="proc ready") -> ("error out"=w175:errorcluster)  [unwired: 8 in, 1 out]
        n169 = local write "error out"(w175) -> ()
      }
      event "qwtb alg params": Mouse Up {
        # "update QWTB parameter info"
        n170 = event-data() -> ()  [unwired: 1 in, 8 out]
        n171 = local read "session out"() -> (w199:T4)
        n172 = control-ref of="qwtb alg params"() -> (w197:refnum<vi>)
        n173 = call "Meas Proc QWTB Get Input Parameter Info.vi"("param table ref"=w197, "session in"=w199) -> ("error out"=w195:errorcluster, "parameter description"=w196:string, "session out"=w198:T4)  [unwired: 7 in]
        n174 = local write "session out"(w198) -> ()
        n175 = local write "qwtb var desc"(w196) -> ()
        n176 = local write "error out"(w195) -> ()
      }
      event "btn qwtb clr params": Value Change {
        # "clear QWTB parameters table"
        n177 = event-data() -> ()  [unwired: 1 in, 6 out]
        n178 = invoke on="qwtb var desc" class="Str" method="Reinit To Default"() -> ()  [unwired: 3 in, 3 out]
        n179 = property on="qwtb alg params" class="Tbl (strict)"("Value"=string[][] [] ("qwtb alg params")) -> ()  [unwired: 2 in, 2 out]
      }
      event "btn mc cfg": Value Change {
        # "QWTB multicore setup"
        n180 = event-data() -> ()  [unwired: 1 in, 6 out]
        n181 = call "SGUI Set Control Enabled State By Groups.vi"("group name to enable (none)"="proc busy") -> ("error out"=w204:errorcluster)  [unwired: 9 in, 1 out]
        n182 = local read "session out"() -> (w207:T4)
        n183 = call "Meas Proc QWTB Multicore Panel.vi"("error in"=w204, "session in"=w207) -> ("error out"=w202:errorcluster, "session out"=w206:T4)  [unwired: 8 in]
        n184 = local write "session out"(w206) -> ()
        n185 = call "SGUI Set Control Enabled State By Groups.vi"("error in"=w202, "group name to enable (none)"="proc ready") -> ("error out"=w201:errorcluster)  [unwired: 8 in, 1 out]
        n186 = local write "error out"(w201) -> ()
      }
      event "btn edit qwtb list": Value Change {
        # "edit qwtb_list.info file"
        n187 = event-data() -> ()  [unwired: 1 in, 6 out]
        n188 = local read "session out"() -> (w209:T4)
        n189 = Unbundle By Name(w209) -> ("processing setup.QWTB.alg filter path"=w208:string)
        n190 = call "Get Root Path.vi"() -> ("root path"=w212:path)
        n191 = Build Path(base path=w212, name or relative path=w208) -> (appended path=w211:path)
        n192 = call "Text Viewer.vi"("Path"=w211) -> ("error out"=w210:errorcluster)  [unwired: 9 in, 1 out]
        n193 = call <vilib>:"Simple Error Handler.vi"("error in (no error)"=w210) -> ()  [unwired: 4 in, 5 out]
      }
      event "qwtb alg params": Shortcut Menu Activation? {
        # "parameters matrix menu"
        n194 = event-data() -> ("CtlRef"=w216:refnum<vi>, "MenuRef"=w217:refnum<k9>, "Coords"=w218:T116)  [unwired: 1 in, 4 out]
        n195 = local read "algorithm info"() -> (w214:T1)
        n196 = Unbundle By Name(w214) -> ("params"=w213:T3[])
        n197 = call "Parameter Matrix Handler.vi"("Operation (Initialization)"=Parameter_Matrix_Operation.vi."On Menu Drop", "matrix reference"=w216, "Mouse Point"=w218, "menu reference"=w217, "parameters"=w213) -> ()  [unwired: 3 in, 4 out]
        n198 = event-data() -> ()  [unwired: 2 in, 1 out]
      }
      event "qwtb alg params": Shortcut Menu Selection (User) {
        # "parameters matrix menu selection made"
        n199 = event-data() -> ("CtlRef"=w223:refnum<vi>, "ItemTag"=w219:string)  [unwired: 1 in, 6 out]
        n200 = local read "algorithm info"() -> (w221:T1)
        n201 = Unbundle By Name(w221) -> ("params"=w220:T3[])
        n202 = call "Parameter Matrix Handler.vi"("Operation (Initialization)"=Parameter_Matrix_Operation.vi."On Menu Select", "menu tag"=w219, "matrix reference"=w223, "parameters"=w220) -> ()  [unwired: 4 in, 4 out]
      }
    }
  }
  n203 = flat-sequence {
    tunnel: w40 -> [_]
    tunnel: w34 -> [w227]
    tunnel: w25 -> [w224]
    frame #0 {
      w225 = SGUI_Assign_References_Mode."Release ID" ("register mode (overwrite)")
      # "on exit action - release GUI controls"
      n204 = call "SGUI Register Controls.vi"("register mode (overwrite)"=w225, "controls ID (empty)"=w227) -> ("error out"=w226:errorcluster)  [unwired: 15 in, 2 out]
      n205 = call "SGUI Register Controls Groups.vi"("error in"=w226, "register mode (overwrite)"=w225, "controls ID (empty)"=w224) -> ()  [unwired: 15 in, 2 out]
      n206 = call <vilib>:"Clear Errors.vi"() -> ()  [unwired: 6 in, 2 out]
    }
  }
  "algorithm info" <- T1 {"name"="", "description"="", "citation"="", "remark"="", "license"="", "description+outs"="", "outputs"=[], "params"=[]} ("algorithm info")
